vi "XW angle calib checker_Psi_STD_PN.vi"(0 "XW_Calib_Map file path (dialog if empty)":path=path "C:/Documents and Settings/Paul Nathan/Desktop/XW Calib Map/XW angle calib checker/XW002_OH74.txt") -> (2 "Quantities that vary with Uref (epsilon, theta, k) (standard method)":string="Uref (m/s)\teps1 (deg)\teps2 (deg)\tProbe zero err. (deg)\ttheta 1 (deg)\ttheta 2 (deg)\r\n0.5018157894736842\t9.3017890724801830\t-6.2576200383800815\t1.5220845170500508\t-30.2854646617259924\t38.4907443143961103\r\n0.9994315789473684\t-0.5078267063761874\t0.4756008610831978\t-0.0161129226464948\t-33.2549649340571562\t37.2028076780815198\r\n2.0002052631578948\t-0.0170670287325283\t0.4389133857835795\t0.2109231785255256\t-40.3150704772274295\t40.5384275834816208\r\n3.0007842105263158\t0.5397928552976248\t-0.1673075851488837\t0.1862426350743706\t-41.7471477428440920\t42.7336376551682235\r\n3.9999473684210529\t0.5552032611501811\t-0.4809296208955749\t0.0371368201273031\t-42.3649922651800707\t43.4904856798574783\r\n4.9998315789473686\t0.5839145398374913\t-0.4879117310338565\t0.0480014044018174\t-42.5176867926462378\t43.6855272441884636\r\n6.9997315789473680\t0.4769954292660519\t-0.3766339827294708\t0.0501807232682906\t-42.6403950914849332\t43.8399700483001169\r\n9.0019315789473691\t0.2955464302508806\t-0.1481957767585597\t0.0736753267461604\t-42.6422862340712001\t43.6715341103828791\r\n10.9999736842105253\t0.0708841951620765\t0.2586334095830275\t0.1647588023725520\t-42.4997912977266665\t43.2532991548099801\r\n13.0001684210526314\t-0.2243455550085545\t0.5043620030432825\t0.1400082240173640\t-42.3214463588717393\t42.9148784991085179\r\n15.0011421052631579\t-0.4668513181945785\t0.7171710888419789\t0.1251598853237002\t-42.1380350724668275\t42.7497636859784933\r\n")   [LabVIEW 2011]
uses:
  <vilib>/Utility/file.llb/Read From Spreadsheet File (DBL).vi
  <vilib>/Utility/file.llb/Read From Spreadsheet File (string).vi
  <vilib>/Analysis/NI_AALPro.lvlib
  <vilib>/Analysis/NI_AALBase.lvlib
panel:
  in  "Ignore first n pts from calib.":i32
  out "Standard effective angle method X plot data (each angle set separated by a column of zeros)":string="x_0\ty1_0\ty2_0\t\tx_1\ty1_1\ty2_1\t\tx_2\ty1_2\ty2_2\t\tx_3\ty1_3\ty2_3\t\tx_4\ty1_4\ty2_4\t\tx_5\ty1_5\ty2_5\t\tx_6\ty1_6\ty2_6\t\tx_7\ty1_7\ty2_7\t\tx_8\ty1_8\ty2_8\t\tx_9\ty1_9\ty2_9\t\tx_10\ty1_10\ty2_10\r\n-0.9999999999999999\t-0.3815133550763904\t-1.2277896709808682\t0.0000000000000000\t-0.9999999999999999\t0.1027343623190909\t-0.9114562899981703\t0.0000000000000000\t-0.9999999999999999\t0.3063443292284778\t-0.9263298161188739\t0.0000000000000000\t-0.9999999999999999\t0.3759098795463195\t-0.9486450743962725\t0.0000000000000000\t-0.9999999999999999\t0.4095937180643089\t-0.9589550813083074\t0.0000000000000000\t-0.9999999999999999\t0.4296105414451811\t-0.9597180393827375\t0.0000000000000000\t-0.9999999999999999\t0.4600573554441755\t-0.9502798289606784\t0.0000000000000000\t-0.9999999999999999\t0.4865160575694266\t-0.9444839218816277\t0.0000000000000000\t-0.9999999999999999\t0.5122386804119141\t-0.9310235854433639\t0.0000000000000000\t-0.9999999999999999\t0.5375704300049343\t-0.9198109803207908\t0.0000000000000000\t-0.9999999999999999\t0.5591838915563910\t-0.9118179530499936\t0.0000000000000000\r\n-0.8459634362504808\t-0.2093643431183902\t-0.9702353019573543\t0.0000000000000000\t-0.8459634362504808\t0.1524007163841222\t-0.7718634095908468\t0.0000000000000000\t-0.8459634362504808\t0.3312481602170517\t-0.7979083840543126\t0.0000000000000000\t-0.8459634362504808\t0.3985703678969933\t-0.8073687738154385\t0.0000000000000000\t-0.8459634362504808\t0.4333153200417899\t-0.8122463376207405\t0.0000000000000000\t-0.8459634362504808\t0.4549729292622101\t-0.8132539080775948\t0.0000000000000000\t-0.8459634362504808\t0.4862152698857382\t-0.8062936170337284\t0.0000000000000000\t-0.8459634362504808\t0.5118762167416807\t-0.8004699517004846\t0.0000000000000000\t-0.8432720672116305\t0.5357418679885581\t-0.7857103524771601\t0.0000000000000000\t-0.8432720672116305\t0.5570613988735588\t-0.7750575851915775\t0.0000000000000000\t-0.8432720672116305\t0.5752714536243961\t-0.7687442796474347\t0.0000000000000000\r\n-0.7028117712403573\t-0.0328228301303722\t-0.6730378859119317\t0.0000000000000000\t-0.7028117712403573\t0.1882864654777492\t-0.6382266361222080\t0.0000000000000000\t-0.7028117712403573\t0.3538653960982250\t-0.6410572155338587\t0.0000000000000000\t-0.7028117712403573\t0.4040956419437625\t-0.6680977866969731\t0.0000000000000000\t-0.7028117712403573\t0.4352309350879587\t-0.6764561489379372\t0.0000000000000000\t-0.7028117712403573\t0.4560210940858728\t-0.6766213078456130\t0.0000000000000000\t-0.7028117712403573\t0.4844463111444350\t-0.6712058868596205\t0.0000000000000000\t-0.7028117712403573\t0.5050363372082499\t-0.6660403761493522\t0.0000000000000000\t-0.7028117712403573\t0.5215750025874688\t-0.6548182695443805\t0.0000000000000000\t-0.7028117712403573\t0.5360488120239911\t-0.6445561268834644\t0.0000000000000000\t-0.7028117712403573\t0.5481371262887226\t-0.6388980385240232\t0.0000000000000000\r\n-0.5745611109571804\t-0.0186406617106857\t-0.5952034519702041\t0.0000000000000000\t-0.5745611109571804\t0.1999513083746903\t-0.5316352108933271\t0.0000000000000000\t-0.5745611109571804\t0.3408985513360128\t-0.5349167839293223\t0.0000000000000000\t-0.5745611109571804\t0.3874531648602888\t-0.5465000145751649\t0.0000000000000000\t-0.5745611109571804\t0.4129373646503266\t-0.5523222557772299\t0.0000000000000000\t-0.5745611109571804\t0.4286042789167682\t-0.5528069650646648\t0.0000000000000000\t-0.5745611109571804\t0.4476788261076887\t-0.5513628506497092\t0.0000000000000000\t-0.5745611109571804\t0.4619956964268012\t-0.5442667592222343\t0.0000000000000000\t-0.5745611109571804\t0.4726441131254100\t-0.5344097418995096\t0.0000000000000000\t-0.5766523484064272\t0.4813401461691441\t-0.5266279420566395\t0.0000000000000000\t-0.5745611109571804\t0.4886114157092954\t-0.5198390729242247\t0.0000000000000000\r\n-0.4610063144273182\t0.0208636190821711\t-0.4490649036536395\t0.0000000000000000\t-0.4610063144273182\t0.2107116811955977\t-0.4068646001903803\t0.0000000000000000\t-0.4610063144273182\t0.3193395628632208\t-0.4184437337601838\t0.0000000000000000\t-0.4610063144273182\t0.3476067541187934\t-0.4413258534669730\t0.0000000000000000\t-0.4610063144273182\t0.3659615795589626\t-0.4470559836159407\t0.0000000000000000\t-0.4667326950738877\t0.3768063206397253\t-0.4473597048819011\t0.0000000000000000\t-0.4610063144273182\t0.3900255577692402\t-0.4431816758867931\t0.0000000000000000\t-0.4610063144273182\t0.3980910606014888\t-0.4381800765192558\t0.0000000000000000\t-0.4610063144273182\t0.4044180258399097\t-0.4282374300168551\t0.0000000000000000\t-0.4629123289077153\t0.4101583924636033\t-0.4212094225246056\t0.0000000000000000\t-0.4629123289077153\t0.4144611423251504\t-0.4160205988735473\t0.0000000000000000\r\n-0.3689194771098271\t0.0536561800579369\t-0.3205162913955928\t0.0000000000000000\t-0.3689194771098271\t0.2064815177911305\t-0.3062154711050765\t0.0000000000000000\t-0.3689194771098271\t0.2799269036558585\t-0.3330488687483389\t0.0000000000000000\t-0.3689194771098271\t0.2991867707938265\t-0.3494639593590201\t0.0000000000000000\t-0.3635749763519443\t0.3117719154399675\t-0.3521145995133866\t0.0000000000000000\t-0.3689194771098271\t0.3167405171150758\t-0.3586129042485994\t0.0000000000000000\t-0.3689194771098271\t0.3245127738637020\t-0.3562226869399766\t0.0000000000000000\t-0.3689194771098271\t0.3292990841472899\t-0.3508926675323383\t0.0000000000000000\t-0.3689194771098271\t0.3339084930327397\t-0.3416397395803143\t0.0000000000000000\t-0.3689194771098271\t0.3384811057696974\t-0.3342993362304802\t0.0000000000000000\t-0.3689194771098271\t0.3420929435861684\t-0.3304456161250302\t0.0000000000000000\r\n-0.2718814121476857\t0.0128752726903403\t-0.2918882287416100\t0.0000000000000000\t-0.2718814121476857\t0.1697376633133504\t-0.2266806671812408\t0.0000000000000000\t-0.2718814121476857\t0.2229566711987844\t-0.2428262977232454\t0.0000000000000000\t-0.2718814121476857\t0.2307298756899231\t-0.2616149044401169\t0.0000000000000000\t-0.2718814121476857\t0.2378391151339257\t-0.2642740709057536\t0.0000000000000000\t-0.2718814121476857\t0.2412383560156202\t-0.2663561249281411\t0.0000000000000000\t-0.2718814121476857\t0.2442971723726146\t-0.2653763300549608\t0.0000000000000000\t-0.2718814121476857\t0.2479980197330459\t-0.2603824415827295\t0.0000000000000000\t-0.2718814121476857\t0.2521992515701980\t-0.2516942950270311\t0.0000000000000000\t-0.2718814121476857\t0.2561334149269846\t-0.2454443997906341\t0.0000000000000000\t-0.2718814121476857\t0.2593097454420143\t-0.2408007167960739\t0.0000000000000000\r\n-0.1761470268806888\t-0.0460636059230048\t-0.2597206147786703\t0.0000000000000000\t-0.1761470268806888\t0.1367610417356654\t-0.1245217926281068\t0.0000000000000000\t-0.1761470268806888\t0.1648204978101121\t-0.1367476713685922\t0.0000000000000000\t-0.1761470268806888\t0.1556324778511593\t-0.1619004749232093\t0.0000000000000000\t-0.1761470268806888\t0.1532471169414098\t-0.1759448683738918\t0.0000000000000000\t-0.1761470268806888\t0.1547459389933540\t-0.1751181415129130\t0.0000000000000000\t-0.1761470268806888\t0.1564743623124086\t-0.1746920439546165\t0.0000000000000000\t-0.1761470268806888\t0.1591965698399837\t-0.1704341495334744\t0.0000000000000000\t-0.1761470268806888\t0.1628768138501873\t-0.1636926807243563\t0.0000000000000000\t-0.1761470268806888\t0.1668358047330725\t-0.1579627379435780\t0.0000000000000000\t-0.1761470268806888\t0.1700148572265357\t-0.1541486543885721\t0.0000000000000000\r\n-0.0850270210113130\t-0.0249192675646609\t-0.1303094859974098\t0.0000000000000000\t-0.0850270210113130\t0.0909442911360152\t-0.0372283574450995\t0.0000000000000000\t-0.0850270210113130\t0.0904809569960206\t-0.0547255925362277\t0.0000000000000000\t-0.0850270210113130\t0.0725065349820468\t-0.0775788408363293\t0.0000000000000000\t-0.0850270210113130\t0.0707041582222505\t-0.0864608498606846\t0.0000000000000000\t-0.0850270210113130\t0.0688797622803253\t-0.0884108632923820\t0.0000000000000000\t-0.0850270210113130\t0.0692035711225545\t-0.0890153288541087\t0.0000000000000000\t-0.0850270210113130\t0.0721708211052060\t-0.0853122198092176\t0.0000000000000000\t-0.0881921819968595\t0.0763170203287837\t-0.0800059689104619\t0.0000000000000000\t-0.0850270210113130\t0.0798388699423815\t-0.0741348845468330\t0.0000000000000000\t-0.0850270210113130\t0.0836442245073950\t-0.0708087068813914\t0.0000000000000000\r\n0.0000000000000000\t-0.0675558762158115\t-0.0721731620420199\t0.0000000000000000\t0.0000000000000000\t0.0521285968471978\t0.0502583416112362\t0.0000000000000000\t0.0000000000000000\t0.0245879588335671\t0.0279813221883405\t0.0000000000000000\t0.0000000000000000\t0.0019621543550413\t0.0050524396498774\t0.0000000000000000\t0.0000000000000000\t-0.0061696027461181\t-0.0061336357868599\t0.0000000000000000\t0.0000000000000000\t-0.0079100013774912\t-0.0085831974669353\t0.0000000000000000\t0.0000000000000000\t-0.0092384175668538\t-0.0101470822923124\t0.0000000000000000\t0.0000000000000000\t-0.0058391003146520\t-0.0072305995118944\t0.0000000000000000\t-0.0015707976187244\t-0.0017088375061246\t-0.0013002294895013\t0.0000000000000000\t0.0000000000000000\t0.0025778929547452\t0.0031882984899375\t0.0000000000000000\t0.0000000000000000\t0.0059712002481367\t0.0057833454771090\t0.0000000000000000\r\n0.0834450784477064\t-0.0206688109096341\t0.0700768572776769\t0.0000000000000000\t0.0834450784477064\t-0.0380941445743377\t0.0872215566308192\t0.0000000000000000\t0.0834450784477064\t-0.0558300201561846\t0.0957331804870974\t0.0000000000000000\t0.0834450784477064\t-0.0732236364720010\t0.0844087191234334\t0.0000000000000000\t0.0834450784477064\t-0.0805173457914918\t0.0736266135577358\t0.0000000000000000\t0.0834450784477064\t-0.0836885579377382\t0.0724345450655375\t0.0000000000000000\t0.0834450784477064\t-0.0839188118734830\t0.0730597462104811\t0.0000000000000000\t0.0834450784477064\t-0.0821903512279210\t0.0749842989827523\t0.0000000000000000\t0.0834450784477064\t-0.0784920538300603\t0.0801463326183820\t0.0000000000000000\t0.0834450784477064\t-0.0753121353965432\t0.0831734404720674\t0.0000000000000000\t0.0834450784477064\t-0.0706862143432525\t0.0868041012508523\t0.0000000000000000\r\n0.1745279388943651\t-0.1182326213774142\t0.0808812827908076\t0.0000000000000000\t0.1745279388943651\t-0.0919271315384520\t0.1642626880908670\t0.0000000000000000\t0.1745279388943651\t-0.1453665715699975\t0.1669601598550158\t0.0000000000000000\t0.1745279388943651\t-0.1575424728174603\t0.1658670012193113\t0.0000000000000000\t0.1745279388943651\t-0.1658273926201979\t0.1615407592894643\t0.0000000000000000\t0.1745279388943651\t-0.1672768362680423\t0.1626087309411399\t0.0000000000000000\t0.1745279388943651\t-0.1672965282061860\t0.1626004048596422\t0.0000000000000000\t0.1761470268806888\t-0.1656200455197691\t0.1659240999845745\t0.0000000000000000\t0.1745279388943651\t-0.1613724034206572\t0.1708574854717018\t0.0000000000000000\t0.1745279388943651\t-0.1568032947140209\t0.1734311556843217\t0.0000000000000000\t0.1745279388943651\t-0.1527780087237028\t0.1761932842903005\t0.0000000000000000\r\n0.2701952220731489\t-0.2175225002327688\t0.0880882833404676\t0.0000000000000000\t0.2701952220731489\t-0.1807404869389231\t0.2092665135850209\t0.0000000000000000\t0.2685104627037557\t-0.2297640478487596\t0.2413798476133460\t0.0000000000000000\t0.2685104627037557\t-0.2499086559150384\t0.2463765459722784\t0.0000000000000000\t0.2685104627037557\t-0.2548595624989720\t0.2472367788056693\t0.0000000000000000\t0.2701952220731489\t-0.2554346520944715\t0.2505176934311722\t0.0000000000000000\t0.2701952220731489\t-0.2534578092342684\t0.2558303573682952\t0.0000000000000000\t0.2685104627037557\t-0.2504810077883826\t0.2583845275495908\t0.0000000000000000\t0.2685104627037557\t-0.2462672749482715\t0.2626302182454011\t0.0000000000000000\t0.2685104627037557\t-0.2413982906865207\t0.2650174184090481\t0.0000000000000000\t0.2685104627037557\t-0.2371690244601109\t0.2679163503262259\t0.0000000000000000\r\n0.3635749763519443\t-0.2985516255068020\t0.1021551175866013\t0.0000000000000000\t0.3671359250169842\t-0.2881963140571548\t0.2355391232305545\t0.0000000000000000\t0.3689194771098271\t-0.3439588090465734\t0.2888506647729097\t0.0000000000000000\t0.3671359250169842\t-0.3472355168880212\t0.3169173246505426\t0.0000000000000000\t0.3671359250169842\t-0.3425848839159632\t0.3283457496428495\t0.0000000000000000\t0.3689194771098271\t-0.3464936379774030\t0.3340185912267175\t0.0000000000000000\t0.3671359250169842\t-0.3431723933244590\t0.3409826857640367\t0.0000000000000000\t0.3671359250169842\t-0.3409978692691930\t0.3463523030395692\t0.0000000000000000\t0.3671359250169842\t-0.3356770523259974\t0.3506363783024263\t0.0000000000000000\t0.3671359250169842\t-0.3305529705086716\t0.3531958170313479\t0.0000000000000000\t0.3671359250169842\t-0.3261242050667670\t0.3565157077764454\t0.0000000000000000\r\n0.4629123289077153\t-0.3592753337637767\t0.1188424710682436\t0.0000000000000000\t0.4629123289077153\t-0.3961455582195348\t0.2468551635371455\t0.0000000000000000\t0.4610063144273182\t-0.4078131503047583\t0.3456317153666766\t0.0000000000000000\t0.4610063144273182\t-0.4336613559080322\t0.3719343122276372\t0.0000000000000000\t0.4610063144273182\t-0.4343780811673295\t0.3879270465443606\t0.0000000000000000\t0.4610063144273182\t-0.4337604569437492\t0.3994360003896873\t0.0000000000000000\t0.4610063144273182\t-0.4309855014982744\t0.4109175742066737\t0.0000000000000000\t0.4610063144273182\t-0.4263261298882018\t0.4192184431454539\t0.0000000000000000\t0.4610063144273182\t-0.4214466527152020\t0.4253481186747629\t0.0000000000000000\t0.4610063144273182\t-0.4162217639675419\t0.4289363399657696\t0.0000000000000000\t0.4667326950738877\t-0.4139340426836660\t0.4328083957106452\t0.0000000000000000\r\n0.5724736448682121\t-0.5459556676862879\t0.0524052118044550\t0.0000000000000000\t0.5724736448682121\t-0.4940989912441419\t0.2609468729150842\t0.0000000000000000\t0.5724736448682121\t-0.5244197561131690\t0.3692623500583355\t0.0000000000000000\t0.5724736448682121\t-0.5373997744456009\t0.4160099264706334\t0.0000000000000000\t0.5724736448682121\t-0.5361687971848075\t0.4384875505219825\t0.0000000000000000\t0.5724736448682121\t-0.5389852146215962\t0.4536227533883877\t0.0000000000000000\t0.5724736448682121\t-0.5349671762898730\t0.4733202527071914\t0.0000000000000000\t0.5724736448682121\t-0.5301767836189272\t0.4867374360740118\t0.0000000000000000\t0.5703899296732948\t-0.5232213788139769\t0.4973275945622862\t0.0000000000000000\t0.5703899296732948\t-0.5181423409572335\t0.5040215477815080\t0.0000000000000000\t0.5703899296732948\t-0.5118352135434456\t0.5103153396928193\t0.0000000000000000\r\n0.7004676747806673\t-0.8082412565209017\t-0.0634037590243930\t0.0000000000000000\t0.7004676747806673\t-0.6224259701282654\t0.2509742966933443\t0.0000000000000000\t0.7004676747806673\t-0.6469848704640956\t0.3824537561774100\t0.0000000000000000\t0.7004676747806673\t-0.6585490574246281\t0.4372421879402547\t0.0000000000000000\t0.7004676747806673\t-0.6592779562802864\t0.4661196573958219\t0.0000000000000000\t0.7004676747806673\t-0.6573717343650598\t0.4865668070365429\t0.0000000000000000\t0.6981287310371237\t-0.6529826553528034\t0.5130509121568261\t0.0000000000000000\t0.7004676747806673\t-0.6500174245829644\t0.5332136801039905\t0.0000000000000000\t0.6981287310371237\t-0.6420156948320364\t0.5494356244515167\t0.0000000000000000\t0.6981287310371237\t-0.6365619576849509\t0.5623462399512057\t0.0000000000000000\t0.6981287310371237\t-0.6303593959361240\t0.5739067524799967\t0.0000000000000000\r\n0.8432720672116305\t-0.8003772739772571\t-0.0179307346096546\t0.0000000000000000\t0.8432720672116305\t-0.8186647773910324\t0.1999751424310329\t0.0000000000000000\t0.8432720672116305\t-0.7801983209141452\t0.3767452557595226\t0.0000000000000000\t0.8432720672116305\t-0.7969533344567685\t0.4370136121768726\t0.0000000000000000\t0.8432720672116305\t-0.7950490039806231\t0.4691633420056094\t0.0000000000000000\t0.8379106495048978\t-0.7894034936610645\t0.4921747103907626\t0.0000000000000000\t0.8432720672116305\t-0.7880677689113339\t0.5184543435768094\t0.0000000000000000\t0.8432720672116305\t-0.7838715744675596\t0.5428662493313512\t0.0000000000000000\t0.8432720672116305\t-0.7775617623673021\t0.5646546016505375\t0.0000000000000000\t0.8432720672116305\t-0.7705293094482739\t0.5833766925023012\t0.0000000000000000\t0.8432720672116305\t-0.7641704745902068\t0.6014324072456010\t0.0000000000000000\r\n0.9999999999999999\t-0.9554471203838094\t-0.0858969643511720\t0.0000000000000000\t0.9999999999999999\t-0.9030897757420824\t0.1878781044403217\t0.0000000000000000\t0.9999999999999999\t-0.9404179116719943\t0.3500910830747300\t0.0000000000000000\t0.9999999999999999\t-0.9348029076345258\t0.4232170765432015\t0.0000000000000000\t0.9999999999999999\t-0.9414384556599829\t0.4537858750473681\t0.0000000000000000\t0.9999999999999999\t-0.9399485982004485\t0.4727859980819380\t0.0000000000000000\t0.9999999999999999\t-0.9349851356346648\t0.4953290283469364\t0.0000000000000000\t0.9999999999999999\t-0.9301726666670225\t0.5167867817836591\t0.0000000000000000\t0.9999999999999999\t-0.9224448768682160\t0.5399071976336627\t0.0000000000000000\t0.9999999999999999\t-0.9159353591364442\t0.5618090475012055\t0.0000000000000000\t0.9999999999999999\t-0.9089085884438031\t0.5839375995713647\t0.0000000000000000\r\n"
  out "E1, E2 maps for each method":string="E1' actual data (Volts)\tE2' actual data (Volts)\tE1' eff. angle method (Volts)\tE2' eff. angle method (Volts)\r\n2.3579666669999999\t2.9299833330000000\t2.0395896997665717\t2.9328725567299103\r\n2.3677166669999998\t2.9294583329999999\t2.2229759600321208\t2.9317042465898777\r\n2.4008333330000000\t2.9260500000000000\t2.3377343167669569\t2.9280299068921094\r\n2.4493749999999999\t2.9185666669999999\t2.4252876660973257\t2.9203955354098214\r\n2.5012333330000001\t2.9088250000000002\t2.4933951475581342\t2.9105498564271732\r\n2.5454750000000002\t2.8961416670000002\t2.5444962163141009\t2.8972084895806418\r\n2.5916916670000001\t2.8796666670000000\t2.5932962266712836\t2.8803907042279793\r\n2.6357833330000000\t2.8591916670000002\t2.6365116405011255\t2.8589275557438158\r\n2.6740083330000002\t2.8352249999999999\t2.6734852724476332\t2.8342193226229382\r\n2.7039083330000002\t2.8084750000000001\t2.7033947062654788\t2.8062562148127403\r\n2.7292333329999998\t2.7755916670000000\t2.7285827443609558\t2.7743852739265726\r\n2.7522583329999999\t2.7347416670000002\t2.7519825795542219\t2.7351857769490371\r\n2.7705500000000001\t2.6868083330000001\t2.7707162675015229\t2.6889651205445642\r\n2.7864583330000001\t2.6357333330000001\t2.7869251327715823\t2.6361899851827268\r\n2.7969249999999999\t2.5853166669999998\t2.7982097891734603\t2.5767009830581906\r\n2.8072916669999999\t2.5308250000000001\t2.8076664849362332\t2.5097557370787613\r\n2.8134833330000002\t2.4766949999999999\t2.8133766584614035\t2.4155406964295745\r\n2.8174833330000002\t2.4419083330000002\t2.8170945987406228\t2.2872498626066324\r\n2.8178166670000002\t2.4331749999999999\t2.8171173442379427\t2.0739015043781590\r\n2.3343583330000000\t2.8727916670000000\t2.0239861365087388\t2.8749489876388608\r\n2.3435000000000001\t2.8738916670000001\t2.1975417726471727\t2.8757064602648690\r\n2.3714750000000002\t2.8703249999999998\t2.3064220586468598\t2.8719611509911518\r\n2.4142416670000002\t2.8624833330000001\t2.3880671783238858\t2.8641129706694453\r\n2.4608750000000001\t2.8512000000000000\t2.4528463298915280\t2.8525716099039187\r\n2.5054500000000002\t2.8424999999999998\t2.5043471033652853\t2.8435738132132702\r\n2.5484416670000001\t2.8258666670000001\t2.5500597207993620\t2.8263240004930599\r\n2.5895250000000001\t2.8049416670000000\t2.5903600691464788\t2.8046603519516120\r\n2.6267416670000001\t2.7825500000000001\t2.6262022217331515\t2.7816750997190507\r\n2.6555416670000000\t2.7572416670000002\t2.6552012173959194\t2.7554273967253837\r\n2.6786083330000001\t2.7247833330000000\t2.6777746956268902\t2.7235055578770364\r\n2.7000750000000000\t2.6853333330000000\t2.6998398803254786\t2.6859049900378817\r\n2.7202500000000001\t2.6422333330000001\t2.7204207146156505\t2.6443183476483778\r\n2.7338249999999999\t2.5924333329999998\t2.7342713039074544\t2.5926269166959042\r\n2.7455750000000001\t2.5466750000000000\t2.7460446222696948\t2.5406178579450600\r\n2.7540749999999998\t2.4944783330000000\t2.7540552420019719\t2.4724338067578486\r\n2.7618916670000000\t2.4476916670000000\t2.7615081667655650\t2.3843136301964321\r\n2.7636250000000002\t2.4171916670000000\t2.7630099651968179\t2.2617445111296450\r\n2.7645749999999998\t2.4109500000000001\t2.7636004624758725\t2.0619468018969167\r\n2.3075791670000001\t2.8102583330000002\t2.0089964937990503\t2.8122092391196531\r\n2.3143783330000001\t2.8105000000000002\t2.1692451736672211\t2.8120127420867869\r\n2.3374916670000001\t2.8074750000000002\t2.2713373467921389\t2.8086762219285344\r\n2.3759583329999998\t2.8013416670000000\t2.3502255205959677\t2.8024289706437471\r\n2.4189250000000002\t2.7911000000000001\t2.4115654286773642\t2.7919544624384089\r\n2.4590999999999998\t2.7811166670000000\t2.4580286929991617\t2.7818944687275433\r\n2.4994583330000002\t2.7651666669999999\t2.5012275432366482\t2.7654734346188512\r\n2.5392833330000002\t2.7464333330000001\t2.5403090179369228\t2.7459954718144264\r\n2.5737250000000000\t2.7246416670000002\t2.5726117460105717\t2.7243539042023279\r\n2.6007166669999999\t2.6997666670000000\t2.6000648104747359\t2.6983837450669692\r\n2.6247250000000002\t2.6711583330000002\t2.6244175809892569\t2.6700834472656307\r\n2.6453000000000002\t2.6334916669999999\t2.6451453836987904\t2.6341096641725317\r\n2.6619666670000002\t2.5904416669999999\t2.6621251587267953\t2.5923034812904673\r\n2.6758500000000001\t2.5444249999999999\t2.6762182790962887\t2.5441240150503699\r\n2.6868249999999998\t2.5016850000000002\t2.6872064354138456\t2.4946668887373571\r\n2.6947916670000001\t2.4541700000000000\t2.6947609976576055\t2.4300238165174246\r\n2.7006916670000001\t2.4125916670000000\t2.7002517904340890\t2.3455625120289674\r\n2.7041916669999999\t2.3881000000000001\t2.7032373067701321\t2.2303196121775088\r\n2.7053166670000000\t2.3835083330000000\t2.7041616969929625\t2.0394752588310658\r\n2.2740350000000000\t2.7394500000000002\t1.9888965958821232\t2.7412722941471630\r\n2.2802375000000001\t2.7401583330000001\t2.1343538232445378\t2.7416112881648735\r\n2.2992593330000002\t2.7379166669999999\t2.2315222768149621\t2.7390906730983739\r\n2.3320333330000000\t2.7315749999999999\t2.3047654561740369\t2.7327589710081690\r\n2.3698583329999998\t2.7217166669999999\t2.3617349721094114\t2.7224881664885294\r\n2.4067666669999999\t2.7124750000000000\t2.4052785148382876\t2.7131907748388033\r\n2.4441916670000001\t2.6973583329999999\t2.4455624869313626\t2.6976100087209871\r\n2.4818250000000002\t2.6800666670000002\t2.4827199825730450\t2.6799921215729974\r\n2.5130499999999998\t2.6580416670000000\t2.5127447358120110\t2.6574732242119432\r\n2.5383499999999999\t2.6351333330000002\t2.5380161764700944\t2.6336273176606388\r\n2.5605583329999999\t2.6081249999999998\t2.5602590109407983\t2.6074583357850729\r\n2.5799750000000001\t2.5730083330000002\t2.5800899069953851\t2.5732514851668262\r\n2.5960666670000001\t2.5331666670000001\t2.5961032113458304\t2.5351484025649800\r\n2.6095083330000000\t2.4905450000000000\t2.6094937166066461\t2.4902476478674158\r\n2.6199750000000002\t2.4518916669999999\t2.6201074903450534\t2.4442717013574442\r\n2.6276833329999998\t2.4097916669999999\t2.6274218921703163\t2.3827933491868900\r\n2.6343500000000000\t2.3747750000000001\t2.6335720028504097\t2.3043131243740471\r\n2.6365666669999999\t2.3542083329999999\t2.6352651869411852\t2.1979727469950676\r\n2.6372249999999999\t2.3495416670000000\t2.6355371970178276\t2.0206328722204168\r\n2.2321166670000001\t2.6560999999999999\t1.9684294426581215\t2.6577172178134587\r\n2.2376083329999998\t2.6560333329999999\t2.0973561134959082\t2.6572554096634176\r\n2.2525750000000002\t2.6530250000000000\t2.1846371842787229\t2.6540636420544308\r\n2.2800241670000001\t2.6478999999999999\t2.2513211064978007\t2.6485005413472500\r\n2.3128224999999998\t2.6395000000000000\t2.3039914641539188\t2.6401139175293542\r\n2.3450083330000000\t2.6305749999999999\t2.3433959642607727\t2.6310204924832177\r\n2.3794666670000000\t2.6172666670000000\t2.3807513954922404\t2.6173186526483287\r\n2.4135749999999998\t2.6010249999999999\t2.4146312764018951\t2.6009186884995810\r\n2.4428333329999998\t2.5811833329999998\t2.4426120510207512\t2.5807339797714763\r\n2.4661166670000001\t2.5598083329999999\t2.4656681658104924\t2.5586917381341974\r\n2.4855499999999999\t2.5341833330000001\t2.4855116702976199\t2.5341124751896000\r\n2.5037333330000000\t2.5027591669999998\t2.5036302877301275\t2.5035525237550127\r\n2.5192749999999999\t2.4664025000000001\t2.5194475452450429\t2.4679454296724042\r\n2.5313500000000002\t2.4283833330000002\t2.5312301771259316\t2.4273112969791173\r\n2.5405500000000001\t2.3935749999999998\t2.5399759705665690\t2.3845636520256690\r\n2.5480333329999998\t2.3577916669999999\t2.5470386846550213\t2.3288217599125969\r\n2.5532666669999999\t2.3286416669999999\t2.5517085370270203\t2.2583688271283400\r\n2.5558833330000001\t2.3118500000000002\t2.5539792571543773\t2.1611533926393642\r\n2.5566333330000002\t2.3058500000000000\t2.5542437701077998\t2.0026571628304319\r\n2.1775000000000002\t2.5542500000000001\t1.9415555742813055\t2.5535039822684187\r\n2.1830250000000002\t2.5535416670000002\t2.0515760060873882\t2.5528409488885657\r\n2.1960166669999999\t2.5513249999999998\t2.1280333659204724\t2.5507638268717474\r\n2.2165416670000000\t2.5454166670000000\t2.1862304370459098\t2.5452617839041642\r\n2.2438583329999999\t2.5389666670000000\t2.2312505488906140\t2.5394665711806734\r\n2.2702916670000000\t2.5302500000000001\t2.2675988928831154\t2.5299799511187833\r\n2.2996759999999998\t2.5183249999999999\t2.3008771430343304\t2.5181277072658399\r\n2.3292166669999999\t2.5031358330000000\t2.3304276891400169\t2.5030703779449945\r\n2.3559749999999999\t2.4863166670000001\t2.3562600801360234\t2.4863587655058175\r\n2.3760916669999999\t2.4666950000000001\t2.3764373981884686\t2.4665699031511434\r\n2.3937666670000000\t2.4444666669999999\t2.3940665703904651\t2.4448853889365343\r\n2.4100833330000002\t2.4163500000000000\t2.4101404129061494\t2.4179339823593757\r\n2.4243666670000001\t2.3856666670000002\t2.4241174321996186\t2.3865429877992042\r\n2.4357583329999999\t2.3528916670000002\t2.4352097369385954\t2.3505529974037724\r\n2.4436166670000001\t2.3235916670000001\t2.4423728946928538\t2.3134500463252969\r\n2.4501916669999999\t2.2949333329999999\t2.4482738230449779\t2.2645432104356891\r\n2.4553416669999999\t2.2722166669999999\t2.4531560217556367\t2.2025800770307180\r\n2.4578833329999998\t2.2576166670000002\t2.4546899973480207\t2.1234607436460573\r\n2.4582000000000002\t2.2499500000000001\t2.4547346941160888\t1.9884250641875831\r\n2.1434833329999998\t2.4913675000000000\t1.9237891650455088\t2.4898848249321008\r\n2.1502083330000001\t2.4918591669999999\t2.0237367442566487\t2.4905347357014502\r\n2.1616333330000002\t2.4891800000000002\t2.0932279940783838\t2.4879445898397705\r\n2.1792166669999999\t2.4840724999999999\t2.1468994044775682\t2.4833563160886225\r\n2.2021833329999998\t2.4772233330000000\t2.1893423236250586\t2.4761883316962998\r\n2.2257333330000000\t2.4692133329999999\t2.2235347904198344\t2.4687610929179624\r\n2.2519166670000001\t2.4583266670000001\t2.2522805866379101\t2.4581809347785417\r\n2.2789400000000000\t2.4450916669999998\t2.2797447212212218\t2.4445771039115458\r\n2.3021067500000001\t2.4280249999999999\t2.3027860955210340\t2.4283441322009560\r\n2.3218883330000000\t2.4108833330000001\t2.3224978508706515\t2.4113104571718162\r\n2.3376666670000001\t2.3902916670000001\t2.3384555460351355\t2.3910674240644307\r\n2.3533249999999999\t2.3650166669999999\t2.3534162448591012\t2.3664434690486824\r\n2.3658250000000001\t2.3365333330000002\t2.3650708231710498\t2.3372965993788632\r\n2.3771583330000001\t2.3082500000000001\t2.3766806250384951\t2.3055545058027098\r\n2.3848583329999999\t2.2828416670000000\t2.3831410060243945\t2.2707692559592494\r\n2.3908583330000002\t2.2581416669999999\t2.3890381088767825\t2.2264662201276790\r\n2.3955750000000000\t2.2385083330000000\t2.3926846180386101\t2.1696188438039501\r\n2.3980583329999998\t2.2255333330000000\t2.3943701140777640\t2.0952170088433557\r\n2.3979333330000001\t2.2170083329999999\t2.3938533657737646\t1.9788862042908513\r\n2.1050916669999999\t2.4168500000000002\t1.9127402638136541\t2.4137325334227357\r\n2.1117916669999999\t2.4177083330000002\t1.9958246310782282\t2.4142631644164938\r\n2.1217166669999998\t2.4152583330000001\t2.0560693014720246\t2.4126225577875515\r\n2.1360083329999999\t2.4109500000000001\t2.1030325104939913\t2.4086686900143359\r\n2.1542916669999999\t2.4042833330000000\t2.1400995182298539\t2.4019585171104119\r\n2.1732416670000001\t2.3967083329999999\t2.1684423576164558\t2.3954861010982538\r\n2.1953499999999999\t2.3868499999999999\t2.1951081650589019\t2.3852835091352285\r\n2.2187583329999998\t2.3741666669999999\t2.2207469910199640\t2.3747534114946194\r\n2.2397000000000000\t2.3594166670000001\t2.2409859609023943\t2.3601173617975930\r\n2.2565833330000000\t2.3436249999999998\t2.2587704455430786\t2.3452968066194142\r\n2.2699833329999999\t2.3238916669999998\t2.2717594061651964\t2.3262130662683442\r\n2.2846758330000001\t2.3031166669999998\t2.2856179243336023\t2.3049916291479930\r\n2.2971474999999999\t2.2791250000000001\t2.2963414336278878\t2.2795788112205875\r\n2.3069916670000001\t2.2548499999999998\t2.3044821077412991\t2.2498740226742204\r\n2.3146800000000001\t2.2347333329999999\t2.3117189407415295\t2.2204999766665585\r\n2.3208058330000001\t2.2148750000000001\t2.3172051349855818\t2.1818781755412364\r\n2.3247091670000000\t2.1991000000000001\t2.3201880631609542\t2.1322226322316244\r\n2.3268333330000002\t2.1878750000000000\t2.3210110378067368\t2.0678940799316967\r\n2.3271250000000001\t2.1803583330000000\t2.3217851908992997\t1.9722390346352847\r\n2.0602083329999998\t2.3236666669999999\t1.8945741084460315\t2.3160192660819017\r\n2.0647416669999998\t2.3234916669999999\t1.9579945301777324\t2.3147606361792992\r\n2.0721750000000001\t2.3222749999999999\t2.0085059309727127\t2.3170264818831048\r\n2.0817916670000001\t2.3177083330000001\t2.0454816829280649\t2.3115221438264446\r\n2.0951333330000002\t2.3128166669999999\t2.0780523505434103\t2.3088780631345016\r\n2.1082666670000001\t2.3056999999999999\t2.1007099247871599\t2.3024682957730995\r\n2.1244999999999998\t2.2963916670000000\t2.1227701507283316\t2.2940263188045642\r\n2.1421666670000001\t2.2852583329999998\t2.1452533220281285\t2.2867307510115102\r\n2.1578333330000001\t2.2717583330000002\t2.1613408743870957\t2.2739070639043182\r\n2.1720666670000002\t2.2582416670000001\t2.1765915224451970\t2.2622537562270653\r\n2.1853250000000002\t2.2438083330000000\t2.1879316211980124\t2.2471645887868465\r\n2.1978916669999999\t2.2268249999999998\t2.1983138379371079\t2.2288322881824261\r\n2.2085750000000002\t2.2084250000000001\t2.2082405123256605\t2.2090979552250873\r\n2.2177166669999999\t2.1911749999999999\t2.2130869597131904\t2.1830435817613303\r\n2.2262333330000001\t2.1776583330000001\t2.2238229762489512\t2.1635665646687663\r\n2.2299083330000000\t2.1629583330000002\t2.2247055338315920\t2.1302079651857735\r\n2.2349833330000002\t2.1523083330000001\t2.2283665816600475\t2.0920478960885767\r\n2.2355416670000001\t2.1430333330000000\t2.2280073959394491\t2.0426169279397808\r\n2.2367249999999999\t2.1377166669999998\t2.2268507673957147\t1.9760802393018486\r\n2.0031583330000000\t2.1960250000000001\t1.9019612645998605\t2.1831421859349507\r\n2.0045999999999999\t2.1949000000000001\t1.9319746950658814\t2.1830336647272226\r\n2.0074833330000001\t2.1930499999999999\t1.9584065903439416\t2.1826576229729575\r\n2.0119250000000002\t2.1903666670000002\t1.9801641259671172\t2.1801844568774982\r\n2.0170333330000001\t2.1855416669999999\t2.0000274625477767\t2.1788799536517498\r\n2.0236333329999998\t2.1812083329999998\t2.0162489268636810\t2.1777133679827481\r\n2.0313416670000000\t2.1737250000000001\t2.0286520782094364\t2.1707048282156798\r\n2.0397916669999998\t2.1643750000000002\t2.0419486186959115\t2.1649401743976786\r\n2.0486416670000001\t2.1545083329999999\t2.0529522074309767\t2.1574905104636430\r\n2.0583250000000000\t2.1458750000000002\t2.0651530618072602\t2.1522677806504142\r\n2.0650333330000001\t2.1343250000000000\t2.0666295474425942\t2.1368143195021050\r\n2.0748666670000002\t2.1247666669999998\t2.0773227366920373\t2.1285187336793170\r\n2.0832999999999999\t2.1147499999999999\t2.0823995257905596\t2.1140351068652841\r\n2.0910083330000000\t2.1058833330000000\t2.0849526345171618\t2.0971600975349647\r\n2.0972083330000002\t2.0990750000000000\t2.0864196057127251\t2.0796416941451303\r\n2.1020249999999998\t2.0923416669999999\t2.0890605762920598\t2.0600755150567536\r\n2.1062166670000000\t2.0873249999999999\t2.0896839126202984\t2.0348423236542255\r\n2.1089833329999998\t2.0837249999999998\t2.0845169297931143\t2.0019675828935743\r\n2.1112916670000001\t2.0818833329999999\t2.0896757218574296\t1.9679402695348538\r\n1.9603916669999999\t2.1036166669999998\t1.8934688001273940\t2.0760101295912388\r\n1.9639500000000001\t2.1090666670000000\t1.9150391481407605\t2.0880779278329378\r\n1.9648583330000000\t2.1094166670000001\t1.9375643137532430\t2.1007171609491402\r\n1.9647833330000000\t2.1051083330000000\t1.9452415389350925\t2.0953221654156229\r\n1.9650666670000001\t2.0985000000000000\t1.9550332022470638\t2.0939099746666976\r\n1.9663583330000001\t2.0928749999999998\t1.9642891216107354\t2.0939175677102417\r\n1.9673416669999999\t2.0863999999999998\t1.9652918270304494\t2.0840508359044243\r\n1.9705333330000001\t2.0802000000000000\t1.9665350032635691\t2.0747891686994242\r\n1.9759333330000000\t2.0757916669999998\t1.9782059506058267\t2.0766180654902922\r\n1.9812083330000001\t2.0706166669999999\t1.9826551832974333\t2.0714914989147863\r\n1.9869916670000001\t2.0655083329999999\t1.9974601612851701\t2.0761059125300494\r\n1.9886999999999999\t2.0561500000000001\t1.9923386963545016\t2.0609213301259333\r\n1.9939833330000001\t2.0512166669999998\t1.9916189875950911\t2.0494920321920445\r\n1.9985250000000001\t2.0469833330000000\t1.9922865106934413\t2.0395649531157347\r\n2.0033666669999999\t2.0445500000000001\t1.9955094259535489\t2.0309281417320171\r\n2.0072916670000001\t2.0421833330000001\t1.9882902965039071\t2.0129827696169316\r\n2.0103749999999998\t2.0405666669999998\t1.9777719086080350\t1.9911729128344049\r\n2.0160833330000001\t2.0411750000000000\t1.9882748694566297\t1.9816940824139573\r\n2.0187750000000002\t2.0414916669999998\t1.9863117544070898\t1.9611513314605555\r\n"
  out "E1', E2' map synthesized from effective angle methods LS fits":cluster{dbl[], dbl[]}[](graph)=[{[2.357966667, 2.367716667, 2.400833333, 2.449375, 2.501233333, 2.545475, 2.591691667, 2.635783333, 2.674008333, 2.703908333, 2.729233333, 2.752258333, 2.77055, 2.786458333, 2.796925, 2.807291667, 2.813483333, 2.817483333, 2.817816667, 2.334358333, 2.3435, 2.371475, 2.414241667, 2.460875, 2.50545, 2.548441667, 2.589525, 2.626741667, 2.655541667, 2.678608333, 2.700075, 2.72025, 2.733825, 2.745575, 2.754075, 2.761891667, 2.763625, 2.764575, 2.307579167, 2.314378333, 2.337491667, 2.375958333, 2.418925, 2.4591, 2.499458333, 2.539283333, 2.573725, 2.600716667, 2.624725, 2.6453, 2.661966667, 2.67585, 2.686825, 2.694791667, 2.700691667, 2.704191667, 2.705316667, 2.274035, 2.2802375, 2.299259333, 2.332033333, 2.369858333, 2.406766667, 2.444191667, 2.481825, 2.51305, 2.53835, 2.560558333, 2.579975, 2.596066667, 2.609508333, 2.619975, 2.627683333, 2.63435, 2.636566667, 2.637225, 2.232116667, 2.237608333, 2.252575, 2.280024167, 2.3128225, 2.345008333, 2.379466667, 2.413575, 2.442833333, 2.466116667, 2.48555, 2.503733333, 2.519275, 2.53135, 2.54055, 2.548033333, 2.553266667, 2.555883333, 2.556633333, 2.1775, 2.183025, 2.196016667, 2.216541667, 2.243858333, 2.270291667, 2.299676, 2.329216667, 2.355975, 2.376091667, 2.393766667, 2.410083333, 2.424366667, 2.435758333, 2.443616667, 2.450191667, 2.455341667, 2.457883333, 2.4582, 2.143483333, 2.150208333, 2.161633333, 2.179216667, 2.202183333, 2.225733333, 2.251916667, 2.27894, 2.30210675, 2.321888333, 2.337666667, 2.353325, 2.365825, 2.377158333, 2.384858333, 2.390858333, 2.395575, 2.398058333, 2.397933333, 2.105091667, 2.111791667, 2.121716667, 2.136008333, 2.154291667, 2.173241667, 2.19535, 2.218758333, 2.2397, 2.256583333, 2.269983333, 2.284675833, 2.2971475, 2.306991667, 2.31468, 2.320805833, 2.324709167, 2.326833333, 2.327125, 2.060208333, 2.064741667, 2.072175, 2.081791667, 2.095133333, 2.108266667, 2.1245, 2.142166667, 2.157833333, 2.172066667, 2.185325, 2.197891667, 2.208575, 2.217716667, 2.226233333, 2.229908333, 2.234983333, 2.235541667, 2.236725, 2.003158333, 2.0046, 2.007483333, 2.011925, 2.017033333, 2.023633333, 2.031341667, 2.039791667, 2.048641667, 2.058325, 2.065033333, 2.074866667, 2.0833, 2.091008333, 2.097208333, 2.102025, 2.106216667, 2.108983333, 2.111291667, 1.960391667, 1.96395, 1.964858333, 1.964783333, 1.965066667, 1.966358333, 1.967341667, 1.970533333, 1.975933333, 1.981208333, 1.986991667, 1.9887, 1.993983333, 1.998525, 2.003366667, 2.007291667, 2.010375, 2.016083333, 2.018775], [2.929983333, 2.929458333, 2.92605, 2.918566667, 2.908825, 2.896141667, 2.879666667, 2.859191667, 2.835225, 2.808475, 2.775591667, 2.734741667, 2.686808333, 2.635733333, 2.585316667, 2.530825, 2.476695, 2.441908333, 2.433175, 2.872791667, 2.873891667, 2.870325, 2.862483333, 2.8512, 2.8425, 2.825866667, 2.804941667, 2.78255, 2.757241667, 2.724783333, 2.685333333, 2.642233333, 2.592433333, 2.546675, 2.494478333, 2.447691667, 2.417191667, 2.41095, 2.810258333, 2.8105, 2.807475, 2.801341667, 2.7911, 2.781116667, 2.765166667, 2.746433333, 2.724641667, 2.699766667, 2.671158333, 2.633491667, 2.590441667, 2.544425, 2.501685, 2.45417, 2.412591667, 2.3881, 2.383508333, 2.73945, 2.740158333, 2.737916667, 2.731575, 2.721716667, 2.712475, 2.697358333, 2.680066667, 2.658041667, 2.635133333, 2.608125, 2.573008333, 2.533166667, 2.490545, 2.451891667, 2.409791667, 2.374775, 2.354208333, 2.349541667, 2.6561, 2.656033333, 2.653025, 2.6479, 2.6395, 2.630575, 2.617266667, 2.601025, 2.581183333, 2.559808333, 2.534183333, 2.502759167, 2.4664025, 2.428383333, 2.393575, 2.357791667, 2.328641667, 2.31185, 2.30585, 2.55425, 2.553541667, 2.551325, 2.545416667, 2.538966667, 2.53025, 2.518325, 2.503135833, 2.486316667, 2.466695, 2.444466667, 2.41635, 2.385666667, 2.352891667, 2.323591667, 2.294933333, 2.272216667, 2.257616667, 2.24995, 2.4913675, 2.491859167, 2.48918, 2.4840725, 2.477223333, 2.469213333, 2.458326667, 2.445091667, 2.428025, 2.410883333, 2.390291667, 2.365016667, 2.336533333, 2.30825, 2.282841667, 2.258141667, 2.238508333, 2.225533333, 2.217008333, 2.41685, 2.417708333, 2.415258333, 2.41095, 2.404283333, 2.396708333, 2.38685, 2.374166667, 2.359416667, 2.343625, 2.323891667, 2.303116667, 2.279125, 2.25485, 2.234733333, 2.214875, 2.1991, 2.187875, 2.180358333, 2.323666667, 2.323491667, 2.322275, 2.317708333, 2.312816667, 2.3057, 2.296391667, 2.285258333, 2.271758333, 2.258241667, 2.243808333, 2.226825, 2.208425, 2.191175, 2.177658333, 2.162958333, 2.152308333, 2.143033333, 2.137716667, 2.196025, 2.1949, 2.19305, 2.190366667, 2.185541667, 2.181208333, 2.173725, 2.164375, 2.154508333, 2.145875, 2.134325, 2.124766667, 2.11475, 2.105883333, 2.099075, 2.092341667, 2.087325, 2.083725, 2.081883333, 2.103616667, 2.109066667, 2.109416667, 2.105108333, 2.0985, 2.092875, 2.0864, 2.0802, 2.075791667, 2.070616667, 2.065508333, 2.05615, 2.051216667, 2.046983333, 2.04455, 2.042183333, 2.040566667, 2.041175, 2.041491667]}, {[2.0395896997665717, 2.222975960032121, 2.337734316766957, 2.4252876660973257, 2.493395147558134, 2.544496216314101, 2.5932962266712836, 2.6365116405011255, 2.6734852724476332, 2.703394706265479, 2.728582744360956, 2.751982579554222, 2.770716267501523, 2.7869251327715823, 2.7982097891734603, 2.807666484936233, 2.8133766584614035, 2.817094598740623, 2.8171173442379427, 2.023986136508739, 2.1975417726471727, 2.30642205864686, 2.388067178323886, 2.452846329891528, 2.5043471033652853, 2.550059720799362, 2.5903600691464788, 2.6262022217331515, 2.6552012173959194, 2.67777469562689, 2.6998398803254786, 2.7204207146156505, 2.7342713039074544, 2.746044622269695, 2.754055242001972, 2.761508166765565, 2.763009965196818, 2.7636004624758725, 2.0089964937990503, 2.169245173667221, 2.271337346792139, 2.3502255205959677, 2.4115654286773642, 2.4580286929991617, 2.501227543236648, 2.5403090179369228, 2.5726117460105717, 2.600064810474736, 2.624417580989257, 2.6451453836987904, 2.6621251587267953, 2.6762182790962887, 2.6872064354138456, 2.6947609976576055, 2.700251790434089, 2.703237306770132, 2.7041616969929625, 1.9888965958821232, 2.134353823244538, 2.231522276814962, 2.304765456174037, 2.3617349721094114, 2.4052785148382876, 2.4455624869313626, 2.482719982573045, 2.512744735812011, 2.5380161764700944, 2.5602590109407983, 2.580089906995385, 2.5961032113458304, 2.609493716606646, 2.6201074903450534, 2.6274218921703163, 2.6335720028504097, 2.635265186941185, 2.6355371970178276, 1.9684294426581215, 2.0973561134959082, 2.184637184278723, 2.2513211064978007, 2.3039914641539188, 2.3433959642607727, 2.3807513954922404, 2.414631276401895, 2.442612051020751, 2.4656681658104924, 2.48551167029762, 2.5036302877301275, 2.519447545245043, 2.5312301771259316, 2.539975970566569, 2.5470386846550213, 2.5517085370270203, 2.5539792571543773, 2.5542437701078, 1.9415555742813055, 2.051576006087388, 2.1280333659204724, 2.18623043704591, 2.231250548890614, 2.2675988928831154, 2.3008771430343304, 2.330427689140017, 2.3562600801360234, 2.3764373981884686, 2.394066570390465, 2.4101404129061494, 2.4241174321996186, 2.4352097369385954, 2.442372894692854, 2.448273823044978, 2.4531560217556367, 2.4546899973480207, 2.454734694116089, 1.9237891650455088, 2.0237367442566487, 2.093227994078384, 2.146899404477568, 2.1893423236250587, 2.2235347904198344, 2.25228058663791, 2.279744721221222, 2.302786095521034, 2.3224978508706515, 2.3384555460351355, 2.353416244859101, 2.3650708231710498, 2.376680625038495, 2.3831410060243945, 2.3890381088767825, 2.39268461803861, 2.394370114077764, 2.3938533657737646, 1.9127402638136541, 1.9958246310782282, 2.0560693014720246, 2.1030325104939913, 2.140099518229854, 2.1684423576164558, 2.195108165058902, 2.220746991019964, 2.2409859609023943, 2.2587704455430786, 2.2717594061651964, 2.2856179243336023, 2.296341433627888, 2.304482107741299, 2.3117189407415295, 2.317205134985582, 2.320188063160954, 2.321011037806737, 2.3217851908992997, 1.8945741084460315, 1.9579945301777324, 2.0085059309727127, 2.045481682928065, 2.0780523505434103, 2.10070992478716, 2.1227701507283316, 2.1452533220281285, 2.1613408743870957, 2.176591522445197, 2.1879316211980124, 2.198313837937108, 2.2082405123256605, 2.2130869597131904, 2.223822976248951, 2.224705533831592, 2.2283665816600475, 2.228007395939449, 2.2268507673957147, 1.9019612645998605, 1.9319746950658814, 1.9584065903439416, 1.9801641259671172, 2.0000274625477767, 2.016248926863681, 2.0286520782094364, 2.0419486186959115, 2.0529522074309767, 2.06515306180726, 2.066629547442594, 2.0773227366920373, 2.0823995257905596, 2.084952634517162, 2.086419605712725, 2.0890605762920598, 2.0896839126202984, 2.0845169297931143, 2.0896757218574296, 1.893468800127394, 1.9150391481407605, 1.937564313753243, 1.9452415389350926, 1.9550332022470638, 1.9642891216107354, 1.9652918270304494, 1.9665350032635691, 1.9782059506058267, 1.9826551832974333, 1.9974601612851701, 1.9923386963545016, 1.9916189875950912, 1.9922865106934413, 1.9955094259535489, 1.988290296503907, 1.977771908608035, 1.9882748694566297, 1.9863117544070898], [2.9328725567299103, 2.9317042465898777, 2.9280299068921094, 2.9203955354098214, 2.9105498564271732, 2.897208489580642, 2.8803907042279793, 2.858927555743816, 2.834219322622938, 2.8062562148127403, 2.7743852739265726, 2.735185776949037, 2.688965120544564, 2.636189985182727, 2.5767009830581906, 2.5097557370787613, 2.4155406964295745, 2.2872498626066324, 2.073901504378159, 2.8749489876388608, 2.875706460264869, 2.871961150991152, 2.8641129706694453, 2.8525716099039187, 2.84357381321327, 2.82632400049306, 2.804660351951612, 2.7816750997190507, 2.7554273967253837, 2.7235055578770364, 2.6859049900378817, 2.644318347648378, 2.592626916695904, 2.54061785794506, 2.4724338067578486, 2.384313630196432, 2.261744511129645, 2.0619468018969167, 2.812209239119653, 2.812012742086787, 2.8086762219285344, 2.802428970643747, 2.791954462438409, 2.7818944687275433, 2.765473434618851, 2.7459954718144264, 2.724353904202328, 2.698383745066969, 2.6700834472656307, 2.6341096641725317, 2.5923034812904673, 2.54412401505037, 2.494666888737357, 2.4300238165174246, 2.3455625120289674, 2.230319612177509, 2.039475258831066, 2.741272294147163, 2.7416112881648735, 2.739090673098374, 2.732758971008169, 2.7224881664885294, 2.7131907748388033, 2.697610008720987, 2.6799921215729974, 2.657473224211943, 2.633627317660639, 2.607458335785073, 2.5732514851668262, 2.53514840256498, 2.490247647867416, 2.444271701357444, 2.38279334918689, 2.304313124374047, 2.1979727469950676, 2.0206328722204168, 2.6577172178134587, 2.6572554096634176, 2.654063642054431, 2.64850054134725, 2.640113917529354, 2.6310204924832177, 2.6173186526483287, 2.600918688499581, 2.5807339797714763, 2.5586917381341974, 2.5341124751896, 2.5035525237550127, 2.467945429672404, 2.4273112969791173, 2.384563652025669, 2.328821759912597, 2.25836882712834, 2.1611533926393642, 2.002657162830432, 2.5535039822684187, 2.5528409488885657, 2.5507638268717474, 2.5452617839041642, 2.5394665711806734, 2.5299799511187833, 2.51812770726584, 2.5030703779449945, 2.4863587655058175, 2.4665699031511434, 2.4448853889365343, 2.4179339823593757, 2.386542987799204, 2.3505529974037724, 2.313450046325297, 2.264543210435689, 2.202580077030718, 2.1234607436460573, 1.9884250641875831, 2.489884824932101, 2.4905347357014502, 2.4879445898397705, 2.4833563160886225, 2.4761883316963, 2.4687610929179624, 2.4581809347785417, 2.444577103911546, 2.428344132200956, 2.4113104571718162, 2.3910674240644307, 2.3664434690486824, 2.3372965993788632, 2.30555450580271, 2.2707692559592494, 2.226466220127679, 2.16961884380395, 2.0952170088433557, 1.9788862042908513, 2.4137325334227357, 2.414263164416494, 2.4126225577875515, 2.408668690014336, 2.401958517110412, 2.3954861010982538, 2.3852835091352285, 2.3747534114946194, 2.360117361797593, 2.345296806619414, 2.3262130662683442, 2.304991629147993, 2.2795788112205875, 2.2498740226742204, 2.2204999766665585, 2.1818781755412364, 2.1322226322316244, 2.0678940799316967, 1.9722390346352847, 2.3160192660819017, 2.314760636179299, 2.317026481883105, 2.3115221438264446, 2.3088780631345016, 2.3024682957730995, 2.294026318804564, 2.2867307510115102, 2.273907063904318, 2.2622537562270653, 2.2471645887868466, 2.228832288182426, 2.2090979552250873, 2.1830435817613303, 2.1635665646687663, 2.1302079651857735, 2.0920478960885767, 2.042616927939781, 1.9760802393018486, 2.1831421859349507, 2.1830336647272226, 2.1826576229729575, 2.180184456877498, 2.17887995365175, 2.177713367982748, 2.17070482821568, 2.1649401743976786, 2.157490510463643, 2.1522677806504142, 2.136814319502105, 2.128518733679317, 2.114035106865284, 2.0971600975349647, 2.0796416941451303, 2.0600755150567536, 2.0348423236542255, 2.0019675828935743, 1.9679402695348538, 2.0760101295912388, 2.0880779278329378, 2.10071716094914, 2.095322165415623, 2.0939099746666976, 2.0939175677102417, 2.0840508359044243, 2.074789168699424, 2.076618065490292, 2.0714914989147863, 2.0761059125300494, 2.0609213301259333, 2.0494920321920445, 2.0395649531157347, 2.030928141732017, 2.0129827696169316, 1.991172912834405, 1.9816940824139573, 1.9611513314605555]}]
  out "E1', E2' map coloured by angle set":cluster{dbl[], dbl[]}[](graph)=[{[1.960391667, 1.96395, 1.964858333, 1.964783333, 1.965066667, 1.966358333, 1.967341667, 1.970533333, 1.975933333, 1.981208333, 1.986991667, 1.9887, 1.993983333, 1.998525, 2.003366667, 2.007291667, 2.010375, 2.016083333, 2.018775], [2.103616667, 2.109066667, 2.109416667, 2.105108333, 2.0985, 2.092875, 2.0864, 2.0802, 2.075791667, 2.070616667, 2.065508333, 2.05615, 2.051216667, 2.046983333, 2.04455, 2.042183333, 2.040566667, 2.041175, 2.041491667]}, {[2.003158333, 2.0046, 2.007483333, 2.011925, 2.017033333, 2.023633333, 2.031341667, 2.039791667, 2.048641667, 2.058325, 2.065033333, 2.074866667, 2.0833, 2.091008333, 2.097208333, 2.102025, 2.106216667, 2.108983333, 2.111291667], [2.196025, 2.1949, 2.19305, 2.190366667, 2.185541667, 2.181208333, 2.173725, 2.164375, 2.154508333, 2.145875, 2.134325, 2.124766667, 2.11475, 2.105883333, 2.099075, 2.092341667, 2.087325, 2.083725, 2.081883333]}, {[2.060208333, 2.064741667, 2.072175, 2.081791667, 2.095133333, 2.108266667, 2.1245, 2.142166667, 2.157833333, 2.172066667, 2.185325, 2.197891667, 2.208575, 2.217716667, 2.226233333, 2.229908333, 2.234983333, 2.235541667, 2.236725], [2.323666667, 2.323491667, 2.322275, 2.317708333, 2.312816667, 2.3057, 2.296391667, 2.285258333, 2.271758333, 2.258241667, 2.243808333, 2.226825, 2.208425, 2.191175, 2.177658333, 2.162958333, 2.152308333, 2.143033333, 2.137716667]}, {[2.105091667, 2.111791667, 2.121716667, 2.136008333, 2.154291667, 2.173241667, 2.19535, 2.218758333, 2.2397, 2.256583333, 2.269983333, 2.284675833, 2.2971475, 2.306991667, 2.31468, 2.320805833, 2.324709167, 2.326833333, 2.327125], [2.41685, 2.417708333, 2.415258333, 2.41095, 2.404283333, 2.396708333, 2.38685, 2.374166667, 2.359416667, 2.343625, 2.323891667, 2.303116667, 2.279125, 2.25485, 2.234733333, 2.214875, 2.1991, 2.187875, 2.180358333]}, {[2.143483333, 2.150208333, 2.161633333, 2.179216667, 2.202183333, 2.225733333, 2.251916667, 2.27894, 2.30210675, 2.321888333, 2.337666667, 2.353325, 2.365825, 2.377158333, 2.384858333, 2.390858333, 2.395575, 2.398058333, 2.397933333], [2.4913675, 2.491859167, 2.48918, 2.4840725, 2.477223333, 2.469213333, 2.458326667, 2.445091667, 2.428025, 2.410883333, 2.390291667, 2.365016667, 2.336533333, 2.30825, 2.282841667, 2.258141667, 2.238508333, 2.225533333, 2.217008333]}, {[2.1775, 2.183025, 2.196016667, 2.216541667, 2.243858333, 2.270291667, 2.299676, 2.329216667, 2.355975, 2.376091667, 2.393766667, 2.410083333, 2.424366667, 2.435758333, 2.443616667, 2.450191667, 2.455341667, 2.457883333, 2.4582], [2.55425, 2.553541667, 2.551325, 2.545416667, 2.538966667, 2.53025, 2.518325, 2.503135833, 2.486316667, 2.466695, 2.444466667, 2.41635, 2.385666667, 2.352891667, 2.323591667, 2.294933333, 2.272216667, 2.257616667, 2.24995]}, {[2.232116667, 2.237608333, 2.252575, 2.280024167, 2.3128225, 2.345008333, 2.379466667, 2.413575, 2.442833333, 2.466116667, 2.48555, 2.503733333, 2.519275, 2.53135, 2.54055, 2.548033333, 2.553266667, 2.555883333, 2.556633333], [2.6561, 2.656033333, 2.653025, 2.6479, 2.6395, 2.630575, 2.617266667, 2.601025, 2.581183333, 2.559808333, 2.534183333, 2.502759167, 2.4664025, 2.428383333, 2.393575, 2.357791667, 2.328641667, 2.31185, 2.30585]}, {[2.274035, 2.2802375, 2.299259333, 2.332033333, 2.369858333, 2.406766667, 2.444191667, 2.481825, 2.51305, 2.53835, 2.560558333, 2.579975, 2.596066667, 2.609508333, 2.619975, 2.627683333, 2.63435, 2.636566667, 2.637225], [2.73945, 2.740158333, 2.737916667, 2.731575, 2.721716667, 2.712475, 2.697358333, 2.680066667, 2.658041667, 2.635133333, 2.608125, 2.573008333, 2.533166667, 2.490545, 2.451891667, 2.409791667, 2.374775, 2.354208333, 2.349541667]}, {[2.307579167, 2.314378333, 2.337491667, 2.375958333, 2.418925, 2.4591, 2.499458333, 2.539283333, 2.573725, 2.600716667, 2.624725, 2.6453, 2.661966667, 2.67585, 2.686825, 2.694791667, 2.700691667, 2.704191667, 2.705316667], [2.810258333, 2.8105, 2.807475, 2.801341667, 2.7911, 2.781116667, 2.765166667, 2.746433333, 2.724641667, 2.699766667, 2.671158333, 2.633491667, 2.590441667, 2.544425, 2.501685, 2.45417, 2.412591667, 2.3881, 2.383508333]}, {[2.334358333, 2.3435, 2.371475, 2.414241667, 2.460875, 2.50545, 2.548441667, 2.589525, 2.626741667, 2.655541667, 2.678608333, 2.700075, 2.72025, 2.733825, 2.745575, 2.754075, 2.761891667, 2.763625, 2.764575], [2.872791667, 2.873891667, 2.870325, 2.862483333, 2.8512, 2.8425, 2.825866667, 2.804941667, 2.78255, 2.757241667, 2.724783333, 2.685333333, 2.642233333, 2.592433333, 2.546675, 2.494478333, 2.447691667, 2.417191667, 2.41095]}, {[2.357966667, 2.367716667, 2.400833333, 2.449375, 2.501233333, 2.545475, 2.591691667, 2.635783333, 2.674008333, 2.703908333, 2.729233333, 2.752258333, 2.77055, 2.786458333, 2.796925, 2.807291667, 2.813483333, 2.817483333, 2.817816667], [2.929983333, 2.929458333, 2.92605, 2.918566667, 2.908825, 2.896141667, 2.879666667, 2.859191667, 2.835225, 2.808475, 2.775591667, 2.734741667, 2.686808333, 2.635733333, 2.585316667, 2.530825, 2.476695, 2.441908333, 2.433175]}]
  out "Probe angles traversed in each angle set\n1st index: angle (deg)\n2nd index: angle set":dbl[][](array[numeric])=[[-45.0, -45.0, -45.0, -45.0, -45.0, -45.0, -45.0, -45.0, -45.0, -45.0, -45.0], [-40.23, -40.23, -40.23, -40.23, -40.23, -40.23, -40.23, -40.23, -40.14, -40.14, -40.14], [-35.1, -35.1, -35.1, -35.1, -35.1, -35.1, -35.1, -35.1, -35.1, -35.1, -35.1], [-29.88, -29.88, -29.88, -29.88, -29.88, -29.88, -29.88, -29.88, -29.88, -29.97, -29.88], [-24.75, -24.75, -24.75, -24.75, -24.75, -25.02, -24.75, -24.75, -24.75, -24.84, -24.84], [-20.25, -20.25, -20.25, -20.25, -19.98, -20.25, -20.25, -20.25, -20.25, -20.25, -20.25], [-15.21, -15.21, -15.21, -15.21, -15.21, -15.21, -15.21, -15.21, -15.21, -15.21, -15.21], [-9.99, -9.99, -9.99, -9.99, -9.99, -9.99, -9.99, -9.99, -9.99, -9.99, -9.99], [-4.86, -4.86, -4.86, -4.86, -4.86, -4.86, -4.86, -4.86, -5.04, -4.86, -4.86], [0.0, 0.0, 0.0, 0.0, 0.0, 0.0, 0.0, 0.0, -0.09, 0.0, 0.0], [4.77, 4.77, 4.77, 4.77, 4.77, 4.77, 4.77, 4.77, 4.77, 4.77, 4.77], [9.9, 9.9, 9.9, 9.9, 9.9, 9.9, 9.9, 9.99, 9.9, 9.9, 9.9], [15.12, 15.12, 15.03, 15.03, 15.03, 15.12, 15.12, 15.03, 15.03, 15.03, 15.03], [19.98, 20.16, 20.25, 20.16, 20.16, 20.25, 20.16, 20.16, 20.16, 20.16, 20.16], [24.84, 24.84, 24.75, 24.75, 24.75, 24.75, 24.75, 24.75, 24.75, 24.75, 25.02], [29.79, 29.79, 29.79, 29.79, 29.79, 29.79, 29.79, 29.79, 29.7, 29.7, 29.7], [35.01, 35.01, 35.01, 35.01, 35.01, 35.01, 34.92, 35.01, 34.92, 34.92, 34.92], [40.14, 40.14, 40.14, 40.14, 40.14, 39.96, 40.14, 40.14, 40.14, 40.14, 40.14], [45.0, 45.0, 45.0, 45.0, 45.0, 45.0, 45.0, 45.0, 45.0, 45.0, 45.0]]
  out "Uref associated with each angle set (m/s)":dbl[](array[numeric])=[0.5018157894736842, 0.9994315789473684, 2.000205263157895, 3.000784210526316, 3.999947368421053, 4.999831578947369, 6.999731578947368, 9.001931578947369, 10.999973684210525, 13.000168421052631, 15.001142105263158] format="%#.2f"
  out "Effective angle X plot":cluster{dbl[], dbl[]}[](graph)=[{[-0.9999999999999999, -0.8459634362504808, -0.7028117712403573, -0.5745611109571804, -0.46100631442731815, -0.3689194771098271, -0.2718814121476857, -0.17614702688068878, -0.08502702101131297, 0.0, 0.0834450784477064, 0.17452793889436508, 0.26851046270375567, 0.3689194771098271, 0.46100631442731815, 0.5724736448682121, 0.7004676747806673, 0.8432720672116305, 0.9999999999999999], [0.30634432922847776, 0.33124816021705167, 0.35386539609822504, 0.3408985513360128, 0.31933956286322085, 0.27992690365585854, 0.2229566711987844, 0.1648204978101121, 0.09048095699602061, 0.024587958833567094, -0.05583002015618459, -0.14536657156999755, -0.22976404784875964, -0.3439588090465734, -0.4078131503047583, -0.524419756113169, -0.6469848704640956, -0.7801983209141452, -0.9404179116719943]}, {[-0.9999999999999999, -0.8459634362504808, -0.7028117712403573, -0.5745611109571804, -0.46100631442731815, -0.3689194771098271, -0.2718814121476857, -0.17614702688068878, -0.08502702101131297, 0.0, 0.0834450784477064, 0.17452793889436508, 0.26851046270375567, 0.3689194771098271, 0.46100631442731815, 0.5724736448682121, 0.7004676747806673, 0.8432720672116305, 0.9999999999999999], [-0.9263298161188739, -0.7979083840543126, -0.6410572155338587, -0.5349167839293223, -0.41844373376018384, -0.3330488687483389, -0.2428262977232454, -0.1367476713685922, -0.05472559253622773, 0.027981322188340485, 0.0957331804870974, 0.16696015985501583, 0.24137984761334605, 0.2888506647729097, 0.3456317153666766, 0.3692623500583355, 0.38245375617740995, 0.37674525575952256, 0.35009108307473]}, {[-0.9999999999999999, -0.8459634362504808, -0.7028117712403573, -0.5745611109571804, -0.46100631442731815, -0.3689194771098271, -0.2718814121476857, -0.17614702688068878, -0.08502702101131297, 0.0, 0.0834450784477064, 0.17452793889436508, 0.26851046270375567, 0.3689194771098271, 0.46100631442731815, 0.5724736448682121, 0.7004676747806673, 0.8432720672116305, 0.9999999999999999], [0.8490646106157206, 0.718316555449873, 0.5968077309329735, 0.48794705527528537, 0.3915604023947652, 0.31339600692555414, 0.23102895093559755, 0.14976847367312107, 0.07242473615963936, 0.00025279617886625743, -0.07057637226415707, -0.14788858030398422, -0.2276620568639879, -0.31289041456782163, -0.3910548100370327, -0.48566959703900026, -0.5943124418060763, -0.7155264972549548, -0.848559018257988]}, {[-0.9999999999999999, -0.8459634362504808, -0.7028117712403573, -0.5745611109571804, -0.46100631442731815, -0.3689194771098271, -0.2718814121476857, -0.17614702688068878, -0.08502702101131297, 0.0, 0.0834450784477064, 0.17452793889436508, 0.26851046270375567, 0.3689194771098271, 0.46100631442731815, 0.5724736448682121, 0.7004676747806673, 0.8432720672116305, 0.9999999999999999], [-0.8562957498298522, -0.7233812051257119, -0.5998589847170553, -0.48919449243934415, -0.3912107169489937, -0.3117511408758629, -0.22801926638152503, -0.14541230657563686, -0.06678698672456035, 0.006580839135572939, 0.07858364379248216, 0.15717691172790887, 0.23827223129491767, 0.3249128191470088, 0.40437239522013957, 0.50055494509206, 0.610997997030858, 0.7342205640609676, 0.8694574281009981]}]
  out "Wire angle error with speed":cluster{dbl[], dbl[]}[](graph)=[{[0.5018157894736842, 0.9994315789473684, 2.000205263157895, 3.000784210526316, 3.999947368421053, 4.999831578947369, 6.999731578947368, 9.001931578947369, 10.999973684210525, 13.000168421052631, 15.001142105263158], [9.301789072480183, -0.5078267063761874, -0.017067028732528303, 0.5397928552976248, 0.5552032611501811, 0.5839145398374913, 0.47699542926605193, 0.29554643025088057, 0.07088419516207646, -0.22434555500855446, -0.46685131819457854]}, {[0.5018157894736842, 0.9994315789473684, 2.000205263157895, 3.000784210526316, 3.999947368421053, 4.999831578947369, 6.999731578947368, 9.001931578947369, 10.999973684210525, 13.000168421052631, 15.001142105263158], [-6.2576200383800815, 0.4756008610831978, 0.43891338578357947, -0.1673075851488837, -0.48092962089557495, -0.4879117310338565, -0.3766339827294708, -0.1481957767585597, 0.2586334095830275, 0.5043620030432825, 0.7171710888419789]}]
  out "Effective angle variation with speed":cluster{dbl[], dbl[]}[](graph)=[{[0.5018157894736842, 0.9994315789473684, 2.000205263157895, 3.000784210526316, 3.999947368421053, 4.999831578947369, 6.999731578947368, 9.001931578947369, 10.999973684210525, 13.000168421052631, 15.001142105263158], [-30.285464661725992, -33.254964934057156, -40.31507047722743, -41.74714774284409, -42.36499226518007, -42.51768679264624, -42.64039509148493, -42.6422862340712, -42.49979129772667, -42.32144635887174, -42.13803507246683]}, {[0.5018157894736842, 0.9994315789473684, 2.000205263157895, 3.000784210526316, 3.999947368421053, 4.999831578947369, 6.999731578947368, 9.001931578947369, 10.999973684210525, 13.000168421052631, 15.001142105263158], [38.49074431439611, 37.20280767808152, 40.53842758348162, 42.73363765516822, 43.49048567985748, 43.685527244188464, 43.83997004830012, 43.67153411038288, 43.25329915480998, 42.91487849910852, 42.74976368597849]}]
  out "Probe zero alignment error":cluster{dbl[], dbl[]}(graph)={[0.5018157894736842, 0.9994315789473684, 2.000205263157895, 3.000784210526316, 3.999947368421053, 4.999831578947369, 6.999731578947368, 9.001931578947369, 10.999973684210525, 13.000168421052631, 15.001142105263158], [1.5220845170500508, -0.016112922646494804, 0.21092317852552558, 0.18624263507437055, 0.0371368201273031, 0.04800140440181741, 0.05018072326829057, 0.07367532674616044, 0.16475880237255197, 0.140008224017364, 0.12515988532370018]}
  out "Zero angle calibration coeffs. (King's 1914 law)":T1={"A1"=2.895294801714706, "B1"=1.359762188126494, "n1"=0.4357683216387929, "A2"=3.2944413738572145, "B2"=1.3280301230872396, "n2"=0.4590330236259289}
  in  "No. of pts. about zero angle to make up linear least squares fit (for std. method)":i32=4
  in  "Query set":i32=3
  out "Pts per set":i32=19
  out "Angle sets":i32=11
  # "This vi allows you to inspect the finer details of your angle calibration. You can check the extent of validity of the effective angle method. The probe zero angle alignment error is given graphically, you can then correct the recorded angles in the calibration file by ADDING the value obtained from the graph where the curve has levelled off (which typically occurs at speed > 4m/s. Similarly the effective angle typically becomes constant at speed > 4m/s)."
  # "of"
  # "Paul Nathan 23/02/10"
  # "0. Actual data\n1. Standard effective angle method"
  # "The numerical data for all the standard effective angle method plots is available for copying and pasting into Excel below"
  # "The numerical data for the E1, E2 plane maps (actual data, and synthesis from both effective angle methods) is available for copying and pasting into Excel below"
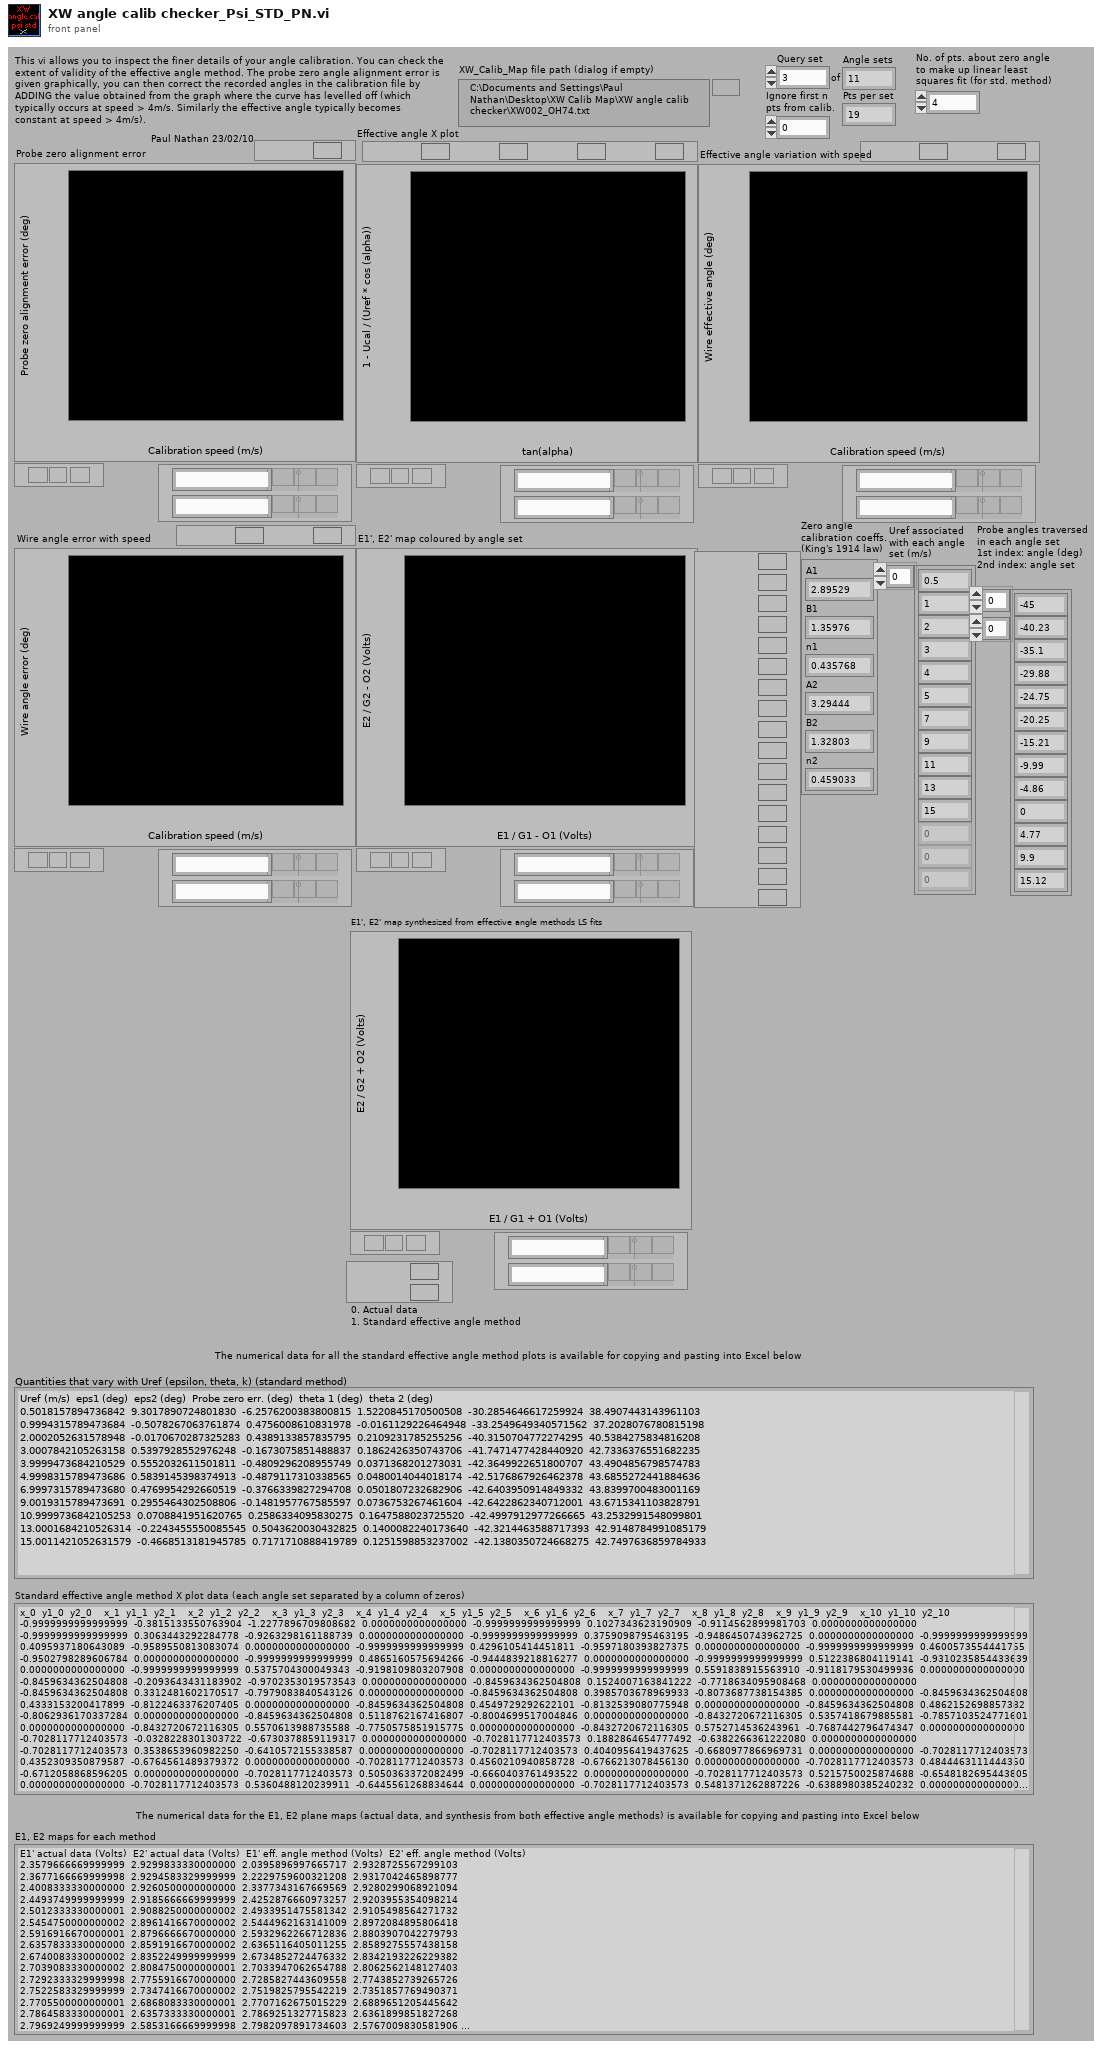
[diagram p1: front panel]
types:
  T1 = cluster{"A1":dbl, "B1":dbl, "n1":dbl, "A2":dbl, "B2":dbl, "n2":dbl}
  T2 = cluster{"A":dbl, "B":dbl, "n":dbl, "A":dbl, "B":dbl, "n":dbl}
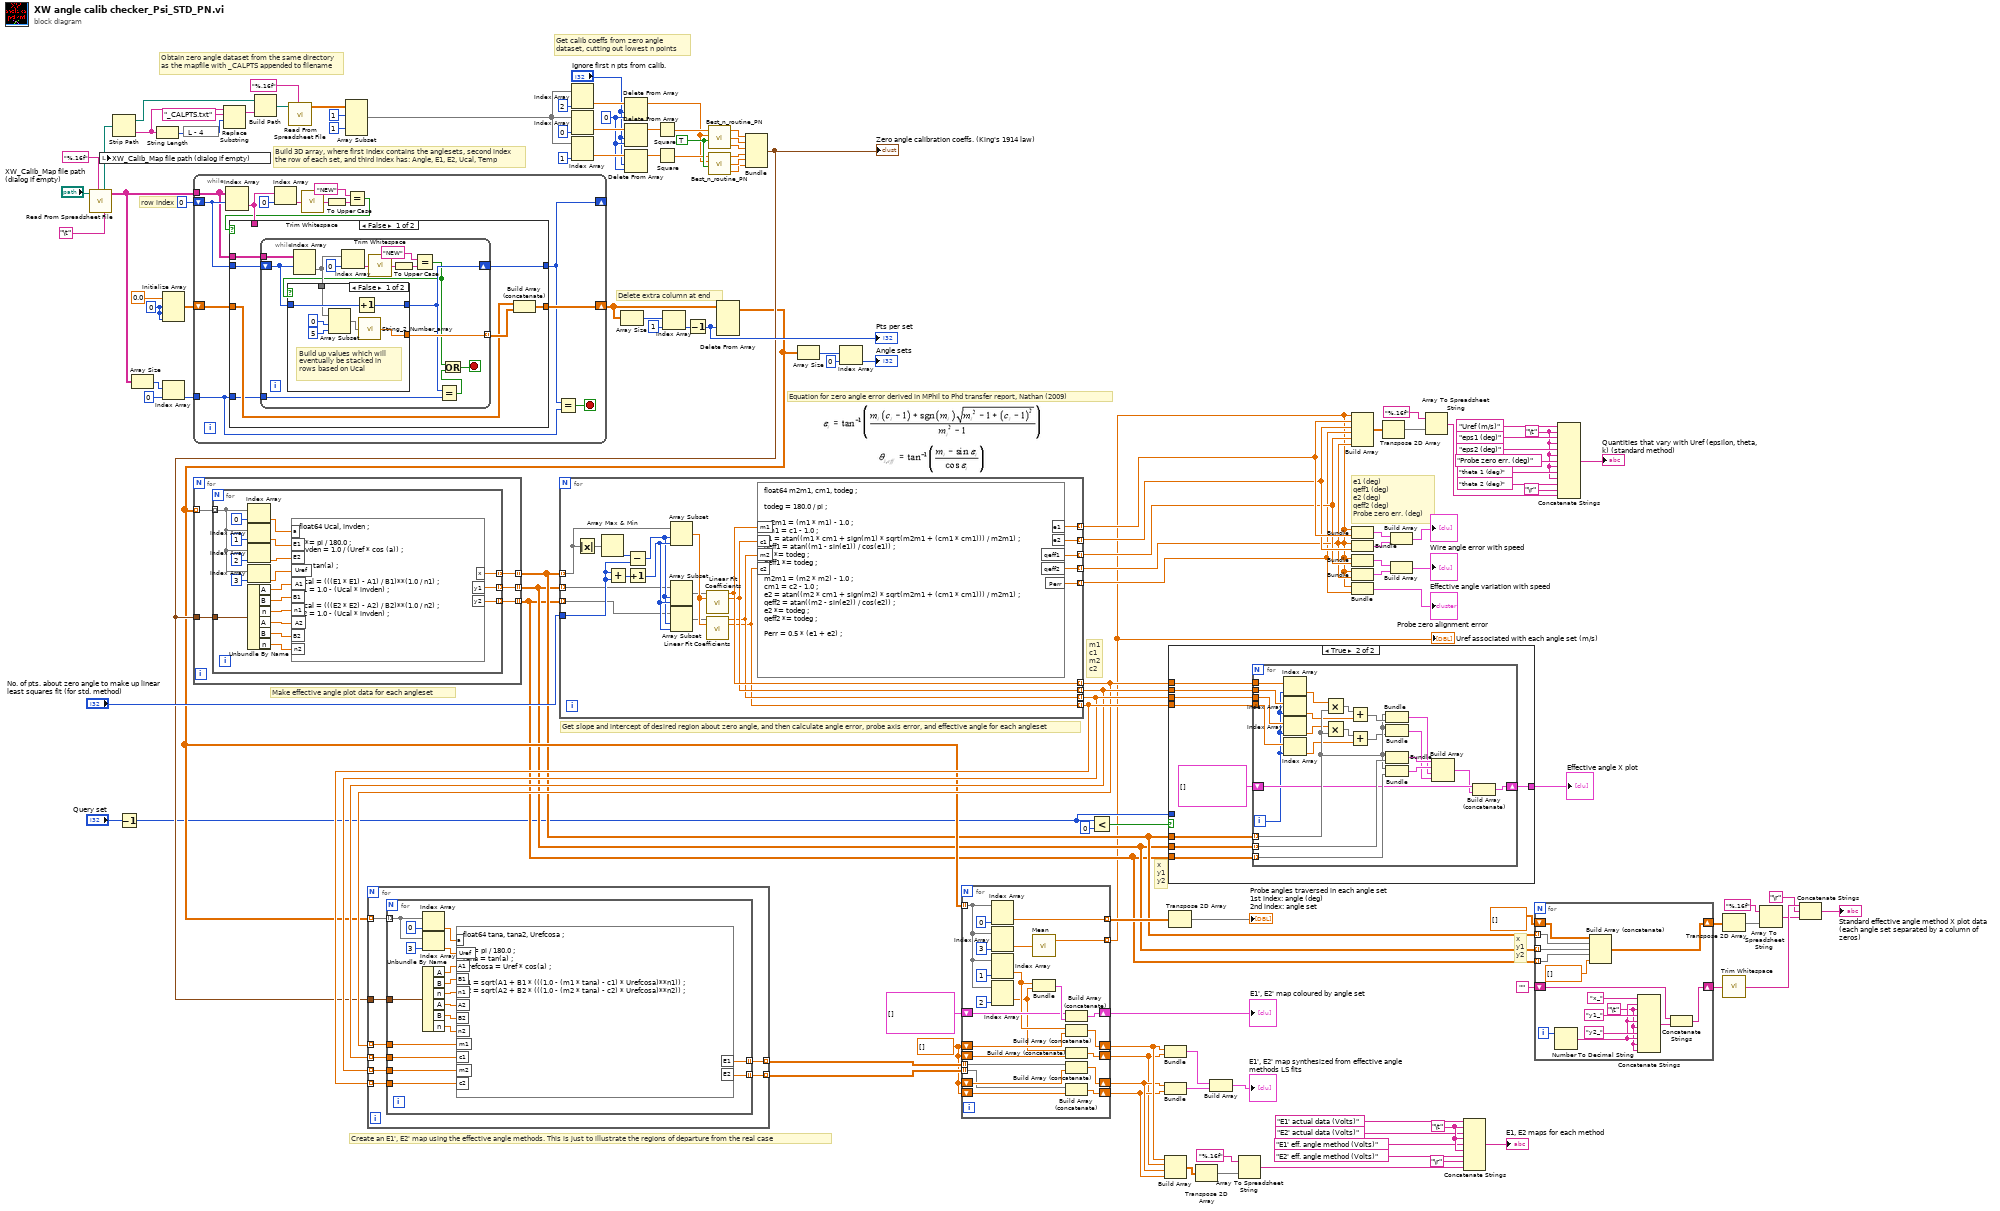
[diagram p0: block diagram]
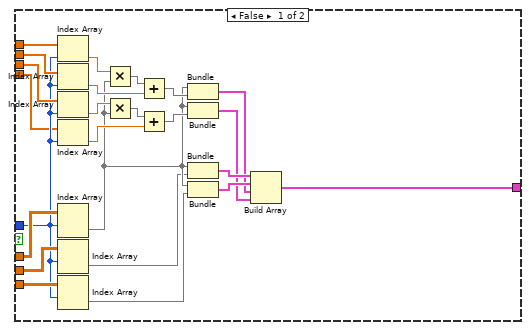
[diagram p2: hidden frame]
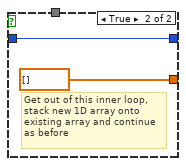
[diagram p3: hidden frame]
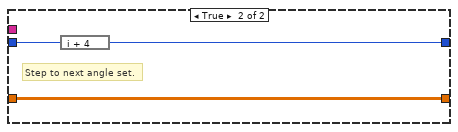
[diagram p4: hidden frame]
diagram:
  w16 = 0 ("index")
  w24 = "\t"
  w53 = "\t"
  w20 = dbl[] []
  w95 = TRUE ("variable n?")
  w112 = 0 ("dimension size")
  # "x\ny1\ny2"
  # "Create an E1', E2' map using the effective angle methods. This is just to illustrate the regions of departure from the real case"
  # "Equation for zero angle error derived in MPhil to Phd transfer report, Nathan (2009)"
  # "x\ny1\ny2"
  # "m1\nc1\nm2\nc2"
  # "e1 (deg)\nqeff1 (deg)\ne2 (deg)\nqeff2 (deg)\nProbe zero err. (deg)"
  # "Get slope and intercept of desired region about zero angle, and then calculate angle error, probe axis error, and effective angle for each angleset"
  # "Make effective angle plot data for each angleset"
  # "Get calib coeffs from zero angle dataset, cutting out lowest n points"
  # "Obtain zero angle dataset from the same directory as the mapfile with _CALPTS appended to filename"
  # "Delete extra column at end"
  # "Build 3D array, where first index contains the anglesets, second index the row of each set, and third index has: Angle, E1, E2, Ucal, Temp"
  # "row index"
  n1 = call-poly <vilib>:"Read From Spreadsheet File.vi"("delimiter (\\t)"="\t", "format (%s)"="%.16f" ("format (%.3f)"), "file path (dialog if empty)"="XW_Calib_Map file path (dialog if empty)") -> ("all rows"=w126:string[][], "new file path (Not A Path if cancelled)"=w98:path)  [unwired: 2 in, 5 out]
  n2 = local write "XW_Calib_Map file path (dialog if empty)"(w98) -> ()
  n3 = Strip Path(path=w98) -> (stripped path=w105:path, name=w109:string)
  n4 = Decrement(x="Query set") -> (x-1=w10:i32)
  n5 = Array Size(array=w126) -> (size(s)=w123:i32[])
  n6 = String Length(string=w109) -> (length=w108:i32)
  n7 = Initialize Array(0.0 ("element"), w112, w112, w112) -> (w111:dbl[][][])
  n8 = Index Array(array=w123, index=0) -> (element=w122:i32)
  n9 = expression code="L - 4"(w108) -> (w107:i32)
  n10 = while {
    tunnel: w126 -> [w135]
    shift-right: [w133] -> w116
    shift-left: w111 -> [w134]
    shift-right: [w132] -> _
    shift-left: 0 ("index") -> [w138]
    tunnel: w122 -> [w131]
    stop <- w140 stop-if-true
    n11 = Index Array(array=w135, index (row)=w138) -> (element=w137:string[])  [unwired: 1 in]
    n12 = Index Array(array=w137, index=0) -> (element=w130:string)
    n13 = call <vilib>:"Trim Whitespace.vi"("string"=w130) -> ("trimmed string"=w129:string)  [unwired: 1 in]
    n14 = To Upper Case(1:w129) -> (0:w142:string)
    n15 = Equal?(x="NEW", y=w142) -> (x = y?=w136:bool)
    n16 = case shown="False" w136 {
      tunnel: w138 -> [w149 w175]
      tunnel: [w144 w173] -> w132
      tunnel: w137 -> [_ _]
      tunnel: w135 -> [w148 _]
      tunnel: w134 -> [w145 w174]
      tunnel: [w147 w174] -> w133
      tunnel: w131 -> [w143 _]
      frame False {
        n17 = while {
          tunnel: w148 -> [w159]
          shift-right: [w154] -> w144
          shift-left: w149 -> [w157]
          tunnel: [w158] -> w146 mode=indexing
          tunnel: w143 -> [w156]
          stop <- w153 stop-if-true
          n18 = Index Array(array=w159, index (row)=w157) -> (element=w160:string[])  [unwired: 1 in]
          n19 = Index Array(array=w160, index=0) -> (element=w151:string)
          n20 = call <vilib>:"Trim Whitespace.vi"("string"=w151) -> ("trimmed string"=w150:string)  [unwired: 1 in]
          n21 = To Upper Case(1:w150) -> (0:w163:string)
          n22 = Equal?(x="NEW", y=w163) -> (x = y?=w152:bool)
          n23 = case shown="False" w152 {
            tunnel: w160 -> [w165 _]
            tunnel: [w164 dbl[] []] -> w158
            tunnel: w157 -> [w168 w172]
            tunnel: [w167 w172] -> w154
            frame False {
              # "Build up values which will eventually be stacked in rows based on Ucal"
              n24 = Array Subset(array=w165, index=0, length=5) -> (w169:string[])
              n25 = Increment(x=w168) -> (x+1=w167:i32)
              n26 = call "String_2_Number_array.vi"("Input String"=w169) -> ("Values"=w164:dbl[])
            }
            frame True {
              # "Get out of this inner loop, stack new 1D array onto existing array and continue as before"
            }
          }
          n27 = Equal?(x=w154, y=w156) -> (x = y?=w155:bool)
          n28 = Or(x=w152, y=w155) -> (x .or. y?=w153:bool)
        }
        n29 = Build Array (concatenate)(w145, w146) -> (w147:dbl[][][])
      }
      frame True {
        # "Step to next angle set."
        n30 = expression code="i + 4"(w175) -> (w173:i32)
      }
    }
    n31 = Equal?(x=w132, y=w131) -> (x = y?=w140:bool)
  }
  n32 = Replace Substring(3:w107, 4:"_CALPTS.txt" ("substring (\"\")"), 5:w109) -> (1:w104:string)  [unwired: 2 out]
  n33 = Build Path(base path=w105, name or relative path=w104) -> (appended path=w99:path)
  n34 = call-poly <vilib>:"Read From Spreadsheet File.vi"("format (%.3f)"="%.16f", "file path (dialog if empty)"=w99) -> ("all rows"=w101:dbl[][])  [unwired: 2 in, 7 out]
  n35 = Array Subset(array=w101, index (row)=1 ("index"), index (col)=1 ("index")) -> (w96:dbl[][])  [unwired: 2 in]
  n36 = Index Array(array=w96, index (col)=2 ("index")) -> (element=w19:dbl[])  [unwired: 1 in]
  n37 = Index Array(array=w96, index (col)=0 ("index")) -> (element=w18:dbl[])  [unwired: 1 in]
  n38 = Index Array(array=w96, index (col)=1 ("index")) -> (element=w17:dbl[])  [unwired: 1 in]
  n39 = Array Size(array=w116) -> (size(s)=w118:i32[])
  n40 = Delete From Array(array=w19, length="Ignore first n pts from calib.", index=w16) -> (array with subset deleted=w15:dbl[])  [unwired: 1 out]
  n41 = Delete From Array(array=w18, length="Ignore first n pts from calib.", index=w16) -> (array with subset deleted=w14:dbl[])  [unwired: 1 out]
  n42 = Delete From Array(array=w17, length="Ignore first n pts from calib.", index=w16) -> (array with subset deleted=w13:dbl[])  [unwired: 1 out]
  n43 = Square(x=w14) -> (x^2=w84:dbl[])
  n44 = Square(x=w13) -> (x^2=w83:dbl[])
  n45 = Index Array(array=w118, index=1) -> (element=w117:i32)
  n46 = Decrement(x=w117) -> (x-1=w114:i32)
  "Pts per set" <- w114
  n47 = call "Best_n_routine_PN.vi"("variable n?"=w95, "U"=w15, "E^2"=w84) -> ("n"=w90:dbl, "B"=w91:dbl, "A"=w92:dbl)  [unwired: 1 in]
  n48 = call "Best_n_routine_PN.vi"("variable n?"=w95, "U"=w15, "E^2"=w83) -> ("n"=w87:dbl, "B"=w88:dbl, "A"=w89:dbl)  [unwired: 1 in]
  n49 = Delete From Array(array=w116, index (dim 1)=w114) -> (array with subset deleted=w60:dbl[][][])  [unwired: 3 in, 1 out]
  n50 = Bundle("A"=w92, "B"=w91, "n"=w90, "A"=w89, "B"=w88, "n"=w87) -> (w61:T2)  [unwired: 1 out]
  "Zero angle calibration coeffs. (King's 1914 law)" <- w61
  n51 = for {
    tunnel: w60 -> [w180] mode=indexing
    tunnel: w61 -> [w179]
    tunnel: [w178] -> w46 mode=indexing
    tunnel: [w177] -> w45 mode=indexing
    tunnel: [w176] -> w44 mode=indexing
    n52 = for {
      tunnel: w180 -> [w185] mode=indexing
      tunnel: w179 -> [w198]
      tunnel: [w183] -> w178 mode=indexing
      tunnel: [w182] -> w177 mode=indexing
      tunnel: [w181] -> w176 mode=indexing
      n53 = Index Array(array=w185, index=0) -> (element=w197:dbl)
      n54 = Index Array(array=w185, index=1) -> (element=w186:dbl)
      n55 = Index Array(array=w185, index=2) -> (element=w184:dbl)
      n56 = Index Array(array=w185, index=3) -> (element=w187:dbl)
      n57 = Unbundle By Name(w198) -> ("A"=w196:dbl, "B"=w195:dbl, "n"=w194:dbl, "A"=w193:dbl, "B"=w192:dbl, "n"=w191:dbl)
      n58 = formula code="float64 Ucal, invden ;\n\na *= pi / 180.0 ;\ninvden = 1.0 / (Uref * cos (a)) ;\n\nx = tan(a) ;\n\nUcal = (((E1 * E1) - A1) / B1)**(1.0 / n1) ;\ny1 = 1.0 - (Ucal * invden) ;\n\nUcal = (((E2 * E2) - A2) / B2)**(1.0 / n2) ;\ny2 = 1.0 - (Ucal * invden) ;"("A1"=w196, "B1"=w195, "n1"=w194, "A2"=w193, "B2"=w192, "n2"=w191, "E1"=w186, "E2"=w184, "a"=w197, "Uref"=w187) -> ("x"=w183:dbl, "y1"=w182:dbl, "y2"=w181:dbl)
    }
  }
  n59 = for {
    tunnel: w46 -> [w219] mode=indexing
    tunnel: w45 -> [w213] mode=indexing
    tunnel: w44 -> [w212] mode=indexing
    tunnel: "No. of pts. about zero angle to make up linear least squares fit (for std. method)" -> [w217]
    tunnel: [w208] -> w9 mode=indexing
    tunnel: [w207] -> w7 mode=indexing
    tunnel: [w206] -> w8 mode=indexing
    tunnel: [w205] -> w6 mode=indexing
    tunnel: [w204] -> w5 mode=indexing
    tunnel: [w203] -> w68 mode=indexing
    tunnel: [w202] -> w69 mode=indexing
    tunnel: [w201] -> w70 mode=indexing
    tunnel: [w200] -> w71 mode=indexing
    n60 = Absolute Value(x=w219) -> (abs(x)=w220:dbl[])
    n61 = Array Max & Min(array=w220) -> (min index (indices)=w218:i32)  [unwired: 3 out]
    n62 = Add(x=w217, y=w217) -> (x+y=w216:i32)
    n63 = Subtract(x=w218, y=w217) -> (x-y=w214:i32)
    n64 = Increment(x=w216) -> (x+1=w215:i32)
    n65 = Array Subset(array=w219, index=w214, length=w215) -> (w211:dbl[])
    n66 = Array Subset(array=w213, index=w214, length=w215) -> (w210:dbl[])
    n67 = Array Subset(array=w212, index=w214, length=w215) -> (w209:dbl[])
    n68 = call <vilib>:"Linear Fit Coefficients.vi"("Y"=w210, "X"=w211) -> ("slope"=w203:dbl, "intercept"=w202:dbl)  [unwired: 3 in, 9 out]
    n69 = call <vilib>:"Linear Fit Coefficients.vi"("Y"=w209, "X"=w211) -> ("slope"=w201:dbl, "intercept"=w200:dbl)  [unwired: 3 in, 9 out]
    n70 = formula code="float64 m2m1, cm1, todeg ;\n\ntodeg = 180.0 / pi ;\n\nm2m1 = (m1 * m1) - 1.0 ;\ncm1 = c1 - 1.0 ;\ne1 = atan((m1 * cm1 + sign(m1) * sqrt(m2m1 + (cm1 * cm1))) / m2m1) ;\nqeff1 = atan((m1 - sin(e1)) / cos(e1)) ;\ne1 *= todeg ;\nqeff1 *= todeg ;\n\nm2m1 = (m2 * m2) - 1.0 ;\ncm1 = c2 - 1.0 ;\ne2 = atan((m2 * cm1 + sign(m2) * sqrt(m2m1 + (cm1 * cm1))) / m2m1) ;\nqeff2 = atan((m2 - sin(e2)) / cos(e2)) ;\ne2 *= todeg ;\nqeff2 *= todeg ;\n\nPerr = 0.5 * (e1 + e2) ;"("m1"=w203, "c1"=w202, "m2"=w201, "c2"=w200) -> ("e1"=w208:dbl, "qeff1"=w207:dbl, "Perr"=w204:dbl, "e2"=w206:dbl, "qeff2"=w205:dbl)
  }
  n71 = for {
    tunnel: w60 -> [w228] mode=indexing
    tunnel: w61 -> [w227]
    tunnel: [w226] -> w66 mode=indexing
    tunnel: [w225] -> w67 mode=indexing
    tunnel: w71 -> [w224] mode=indexing
    tunnel: w70 -> [w223] mode=indexing
    tunnel: w69 -> [w222] mode=indexing
    tunnel: w68 -> [w221] mode=indexing
    n72 = for {
      tunnel: w228 -> [w235] mode=indexing
      tunnel: w227 -> [w245]
      tunnel: [w234] -> w226 mode=indexing
      tunnel: [w233] -> w225 mode=indexing
      tunnel: w224 -> [w232]
      tunnel: w223 -> [w231]
      tunnel: w222 -> [w230]
      tunnel: w221 -> [w229]
      n73 = Index Array(array=w235, index=0) -> (element=w244:dbl)
      n74 = Index Array(array=w235, index=3) -> (element=w236:dbl)
      n75 = Unbundle By Name(w245) -> ("A"=w243:dbl, "B"=w242:dbl, "n"=w241:dbl, "A"=w240:dbl, "B"=w239:dbl, "n"=w238:dbl)
      n76 = formula code="float64 tana, tana2, Urefcosa ;\n\na *= pi / 180.0 ;\ntana = tan(a) ;\nUrefcosa = Uref * cos(a) ;\n\nE1 = sqrt(A1 + B1 * (((1.0 - (m1 * tana) - c1) * Urefcosa)**n1)) ;\nE2 = sqrt(A2 + B2 * (((1.0 - (m2 * tana) - c2) * Urefcosa)**n2)) ;"("A1"=w243, "B1"=w242, "n1"=w241, "A2"=w240, "B2"=w239, "n2"=w238, "a"=w244, "Uref"=w236, "m1"=w229, "c1"=w230, "m2"=w231, "c2"=w232) -> ("E1"=w234:dbl, "E2"=w233:dbl)
    }
  }
  n77 = Array Size(array=w60) -> (size(s)=w121:i32[])
  n78 = Index Array(array=w121, index=0) -> (element=→"Angle sets":i32)
  n79 = for {
    shift-right: [w262] -> w74
    shift-left: cluster{dbl[], dbl[]}[] [] -> [w259]
    tunnel: w60 -> [w263] mode=indexing
    tunnel: [w269] -> w73 mode=indexing
    tunnel: [w267] -> w4 mode=indexing
    shift-right: [w258] -> w57
    shift-left: w20 -> [w253]
    tunnel: w67 -> [w254] mode=indexing
    tunnel: w66 -> [w255] mode=indexing
    shift-right: [w256] -> w58
    shift-left: w20 -> [w257]
    shift-right: [w249] -> w47
    shift-left: w20 -> [w252]
    shift-right: [w251] -> w59
    shift-left: w20 -> [w250]
    n80 = Index Array(array=w263, index (col)=0 ("index")) -> (element=w269:dbl[])  [unwired: 1 in]
    n81 = Index Array(array=w263, index (col)=3 ("index")) -> (element=w268:dbl[])  [unwired: 1 in]
    n82 = Index Array(array=w263, index (col)=1 ("index")) -> (element=w248:dbl[])  [unwired: 1 in]
    n83 = Index Array(array=w263, index (col)=2 ("index")) -> (element=w247:dbl[])  [unwired: 1 in]
    n84 = call <vilib>:"Mean.vi"("X"=w268) -> ("mean"=w267:dbl)  [unwired: 1 out]
    n85 = Bundle(w248, w247) -> (w260:cluster{dbl[], dbl[]})  [unwired: 1 out]
    n86 = Build Array (concatenate)(w259, w260) -> (w262:cluster{dbl[], dbl[]}[])
    n87 = Build Array (concatenate)(w248, w250) -> (w251:dbl[])
    n88 = Build Array (concatenate)(w247, w252) -> (w249:dbl[])
    n89 = Build Array (concatenate)(w255, w257) -> (w256:dbl[])
    n90 = Build Array (concatenate)(w254, w253) -> (w258:dbl[])
  }
  "Uref associated with each angle set (m/s)" <- w4
  "E1', E2' map coloured by angle set" <- w74
  n91 = Less?(x=w10, y=0) -> (x < y?=w11:bool)
  n92 = Bundle(w59, w47) -> (w64:cluster{dbl[], dbl[]})  [unwired: 1 out]
  n93 = Bundle(w58, w57) -> (w63:cluster{dbl[], dbl[]})  [unwired: 1 out]
  n94 = Build Array(w59, w47, w58, w57) -> (w56:dbl[][])
  n95 = case shown="True" w11 {
    tunnel: w68 -> [w290 w299]
    tunnel: w69 -> [w289 w298]
    tunnel: w70 -> [w288 w297]
    tunnel: w71 -> [w286 w296]
    tunnel: w46 -> [w293 w302]
    tunnel: w45 -> [w292 w301]
    tunnel: w44 -> [w291 w300]
    tunnel: [w270 w294] -> w75
    tunnel: w10 -> [w287 _]
    frame False {
      n96 = Index Array(array=w290, index=w287) -> (element=w278:dbl)
      n97 = Index Array(array=w289, index=w287) -> (element=w277:dbl)
      n98 = Index Array(array=w288, index=w287) -> (element=w276:dbl)
      n99 = Index Array(array=w286, index=w287) -> (element=w275:dbl)
      n100 = Index Array(array=w293, index (row)=w287) -> (element=w274:dbl[])  [unwired: 1 in]
      n101 = Index Array(array=w292, index (row)=w287) -> (element=w273:dbl[])  [unwired: 1 in]
      n102 = Index Array(array=w291, index (row)=w287) -> (element=w272:dbl[])  [unwired: 1 in]
      n103 = Multiply(x=w278, y=w274) -> (x*y=w283:dbl[])
      n104 = Multiply(x=w276, y=w274) -> (x*y=w281:dbl[])
      n105 = Add(x=w283, y=w277) -> (x+y=w282:dbl[])
      n106 = Add(x=w281, y=w275) -> (x+y=w280:dbl[])
      n107 = Bundle(w274, w282) -> (w279:cluster{dbl[], dbl[]})  [unwired: 1 out]
      n108 = Bundle(w274, w280) -> (w271:cluster{dbl[], dbl[]})  [unwired: 1 out]
      n109 = Bundle(w274, w273) -> (w285:cluster{dbl[], dbl[]})  [unwired: 1 out]
      n110 = Bundle(w274, w272) -> (w284:cluster{dbl[], dbl[]})  [unwired: 1 out]
      n111 = Build Array(w285, w284, w279, w271) -> (w270:cluster{dbl[], dbl[]}[])
    }
    frame True {
      n112 = for {
        tunnel: w302 -> [w318] mode=indexing
        tunnel: w301 -> [w324] mode=indexing
        tunnel: w300 -> [w322] mode=indexing
        tunnel: w299 -> [w311]
        tunnel: w298 -> [w310]
        tunnel: w297 -> [w309]
        tunnel: w296 -> [w308]
        shift-right: [w312] -> w294
        shift-left: cluster{dbl[], dbl[]}[] [] -> [w314]
        i -> [w307]
        n113 = Index Array(array=w311, index=w307) -> (element=w306:dbl)
        n114 = Index Array(array=w310, index=w307) -> (element=w305:dbl)
        n115 = Index Array(array=w309, index=w307) -> (element=w304:dbl)
        n116 = Index Array(array=w308, index=w307) -> (element=w303:dbl)
        n117 = Multiply(x=w306, y=w318) -> (x*y=w321:dbl[])
        n118 = Multiply(x=w304, y=w318) -> (x*y=w319:dbl[])
        n119 = Add(x=w321, y=w305) -> (x+y=w320:dbl[])
        n120 = Add(x=w319, y=w303) -> (x+y=w317:dbl[])
        n121 = Bundle(w318, w320) -> (w316:cluster{dbl[], dbl[]})  [unwired: 1 out]
        n122 = Bundle(w318, w317) -> (w315:cluster{dbl[], dbl[]})  [unwired: 1 out]
        n123 = Bundle(w318, w324) -> (w325:cluster{dbl[], dbl[]})  [unwired: 1 out]
        n124 = Bundle(w318, w322) -> (w323:cluster{dbl[], dbl[]})  [unwired: 1 out]
        n125 = Build Array(w325, w323, w316, w315) -> (w313:cluster{dbl[], dbl[]}[])
        n126 = Build Array (concatenate)(w314, w313) -> (w312:cluster{dbl[], dbl[]}[])
      }
    }
  }
  "Effective angle X plot" <- w75
  n127 = Transpose 2D Array(2D array=w73) -> (transposed array=→"Probe angles traversed in each angle set\n1st index: angle (deg)\n2nd index: angle set":dbl[][])
  n128 = Transpose 2D Array(2D array=w56) -> (transposed array=w54:dbl[][])
  n129 = Build Array(w64, w63) -> (→"E1', E2' map synthesized from effective angle methods LS fits":cluster{dbl[], dbl[]}[])
  n130 = Array To Spreadsheet String(array=w54, 3:"%.16f" ("format string")) -> (spreadsheet string=w2:string)  [unwired: 1 out]
  n131 = Build Array(w4, w9, w8, w5, w7, w6) -> (w33:dbl[][])
  n132 = Bundle(w4, w9) -> (w79:cluster{dbl[], dbl[]})  [unwired: 1 out]
  n133 = Bundle(w4, w8) -> (w80:cluster{dbl[], dbl[]})  [unwired: 1 out]
  n134 = Bundle(w4, w7) -> (w82:cluster{dbl[], dbl[]})  [unwired: 1 out]
  n135 = Bundle(w4, w6) -> (w81:cluster{dbl[], dbl[]})  [unwired: 1 out]
  n136 = Bundle(w4, w5) -> (→"Probe zero alignment error":cluster{dbl[], dbl[]})  [unwired: 1 out]
  n137 = Transpose 2D Array(2D array=w33) -> (transposed array=w32:dbl[][])
  n138 = Build Array(w79, w80) -> (→"Wire angle error with speed":cluster{dbl[], dbl[]}[])
  n139 = Build Array(w82, w81) -> (→"Effective angle variation with speed":cluster{dbl[], dbl[]}[])
  n140 = Array To Spreadsheet String(array=w32, 3:"%.16f" ("format string")) -> (spreadsheet string=w22:string)  [unwired: 1 out]
  n141 = Concatenate Strings("E1' actual data (Volts)", w53, "E2' actual data (Volts)", w53, "E1' eff. angle method (Volts)", w53, "E2' eff. angle method (Volts)", "\r", w2) -> (→"E1, E2 maps for each method":string)
  n142 = for {
    tunnel: w46 -> [w331] mode=indexing
    tunnel: w45 -> [w330] mode=indexing
    tunnel: w44 -> [w329] mode=indexing
    shift-right: [w334] -> w38
    shift-left: "" -> [w333]
    shift-right: [w327] -> w39
    shift-left: dbl[][] [] -> [w326]
    i -> [w340]
    w335 = "\t"
    n143 = Number To Decimal String(number=w340) -> (decimal integer string=w336:string)  [unwired: 1 out]
    n144 = Build Array (concatenate)(w326, w331, w330, w329, dbl[] [] ("element")) -> (w327:dbl[][])
    n145 = Concatenate Strings("x_" ("format string"), w336, w335, "y1_" ("format string"), w336, w335, "y2_" ("format string"), w336, w335, w335) -> (w332:string)
    n146 = Concatenate Strings(w333, w332) -> (w334:string)
  }
  n147 = Concatenate Strings("Uref (m/s)", w24, "eps1 (deg)", w24, "eps2 (deg)", w24, "Probe zero err. (deg)", w24, "theta 1 (deg)", w24, "theta 2 (deg)", "\r", w22) -> (→"Quantities that vary with Uref (epsilon, theta, k) (standard method)":string)
  n148 = Transpose 2D Array(2D array=w39) -> (transposed array=w41:dbl[][])
  n149 = call <vilib>:"Trim Whitespace.vi"("string"=w38) -> ("trimmed string"=w37:string)  [unwired: 1 in]
  n150 = Array To Spreadsheet String(array=w41, 3:"%.16f" ("format string")) -> (spreadsheet string=w34:string)  [unwired: 1 out]
  n151 = Concatenate Strings(w37, "\r", w34) -> (→"Standard effective angle method X plot data (each angle set separated by a column of zeros)":string)
